vi "why_editsandweird.vi"() -> ()   [LabVIEW 2023]
uses:
  <vilib>/Analysis/NI_AALBase.lvlib
  <vilib>/DAQmx/read.llb/DAQmx Read (Analog 1D DBL NChan 1Samp).vi
  Supporting VIs/Logic states.ctl
  Supporting VIs/Motor states.ctl
  Supporting VIs/Axes indices.ctl
  <instrlib>/Arcus Driver 3.0.0/ArcusUsbComm/classes/Controller/_Controller.lvclass
  <instrlib>/Arcus Driver 3.0.0/ArcusUsbComm/common/controls/linear_direction.ctl
  Supporting VIs/Queue names.ctl
  <vilib>/addons/control/pid/NI_PID_pid.lvlib
  <vilib>/Utility/file.llb/Write Delimited Spreadsheet (string).vi
  <vilib>/Utility/file.llb/Write Delimited Spreadsheet (DBL).vi
  <vilib>/addons/control/pid/pid.llb/PID (DBL).vi
  <vilib>/DAQmx/configure/timing.llb/DAQmx Timing (Sample Clock).vi
  <vilib>/DAQmx/create/channels.llb/DAQmx Create Channel (AI-Voltage-Basic).vi
  <vilib>/Analysis/baseanly.llb/Vector x A.vi
  <vilib>/Analysis/baseanly.llb/A x Vector.vi
  Supporting VIs/Sampling frequency.ctl
panel:
  out "n":dbl format="%#_13g"
  in  "veloincrement":dbl format="%#_13g"
  in  "currentvelo":dbl format="%#_13g"
  in  "min velo":dbl
  in  "max velo":dbl
  in  "no of speedstops":dbl
  out "Steady State COFs":dbl[](array[numeric])
  out "Fixed amplitude Load":dbl(graph)=8.923720573303449
  in  "VISA resource name":refnum<visa-resource-name>
  out "Mean Estimated Friction Coefficient":dbl[](array[numeric])
  in  "Maximum COF Difference":i32=3000
  in  "Number of Previous Points":i32=3000
  out "Torque":dbl(graph)=-1.1532615270996815
  out "Sliding Distance (mm)":i32
  out "Angular Position":dbl
  in  "Initial Position":dbl
  in  "Track Radius (mm)":T1=100 items=["4 mm"=4, "6 mm"=6, "8 mm"=8, "10 mm"=10, "12 mm"=12, "14 mm"=14, "16 mm"=16, "18 mm"=18]
  out "Revolutions Completed":u8(slide) scale=0.0..10.0
  in  "STOP Rotating Motor":bool
  in  "Clockwise":bool
  in  "no of revs per velocity":i32
  out "Progress":dbl(slide) scale=0.0..100.0
  in  "Velocity":dbl
  in  "Units (0: microsteps)":u16(ring) items=["device speed units", "microns per second", "millimeters per second", "inches per second", "degrees per second"]
  in  "Microstep Size (0)":dbl
  in  "Wait [min]":dbl=30.0 format="%.2g"
  in  "Wait ?":bool=TRUE
  in  "Save file name":path=path "C:/Users/Egberts/Desktop/Tribometer/August 2020 Measurements/Tribometer/Late August 2020/test.txt"
  in  "PID gains":T2={"proportional gain (Kc)"=0.02, "integral time (Ti, min)"=0.1, "derivative time (Td, min)"=0.001} {"derivative time (Td, min)" format="%.3f"; "integral time (Ti, min)" format="%.3f"; "proportional gain (Kc)" format="%.3f"}
  in  "output range":cluster{"output high":dbl, "output low":dbl}={"output high"=2.0, "output low"=-2.0} {"output low" format="%.2f"; "output high" format="%.2f"}
  out "x-position":i32
  out "z-position":string
  in  "set zero":bool
  out "Correction loop":i32
  out "received P":i32
  out "Actual Load":dbl
  out "Correction [N]":dbl format="%.2f"
  out "correction [p]":dbl
  out "to PID":i32
  out "dt out (s)":dbl=0.25 format="%.3f"
  in  "Testing Load [N]":dbl=20.0
  in  "Wear cycles":i32=3000
  out "Manual control":bool
  in  "Approach":bool
  in  "DAQmx Device Name":tag="Dev1"
  in  "Out":bool
  in  "In":bool
  in  "Left":bool
  in  "Right":bool
  in  "Up":bool
  out "Estimated friction coefficient":dbl(graph)=-0.11599973982411911
  out "Smooth Force from Torque":dbl(graph)=-1.1532615270996815
  out "Smooth z":dbl(graph)=9.94193201509139
  out "Dequeued Data":dbl[](graph)=[9.378691263157721, 10.717600289594278, 8.438969804942502, 9.318124790458075, 8.681089909963866, 9.970529667476073, 10.834102440336615, 9.183821958337319, 9.334582664259113, 9.226213467034226, 10.238553338370796, 11.173780758664948, 8.690449558950064, 9.261606371512476, 8.790570665988898, 9.887706352746802, 11.038667014275244, 8.916330650848511, 9.104119720861869, 8.923720573303449]
  in  "ABORT":bool
  in  "Down":bool
  out "Aborted":bool
  out "Mean z":dbl[](array[numeric])
  out "Current reading":dbl[](array[numeric])
  in  "Averaging Level":i32=12
  out "Mean Force from Torque":dbl[](array[numeric])
  out "Completed":bool
  out "Testing":bool
  out "Approaching":bool
  in  "TARE":bool
  in  "Sampling frequency (rate)":T1=100 items=["1000 Hz"=1000, " 500 Hz"=500, " 250 Hz"=250, "100 Hz"=100, "50 Hz"=50, "10 Hz"=10, "1 Hz"=1]
  in  "Calibration file":path=path "C:/Users/Egberts/Desktop/ATI Industrial Automation/FT21774.cal"
  # "Counterclockwise"
  # "Originally used to measure \nthe amount of positions needed\nto perform fast approach"
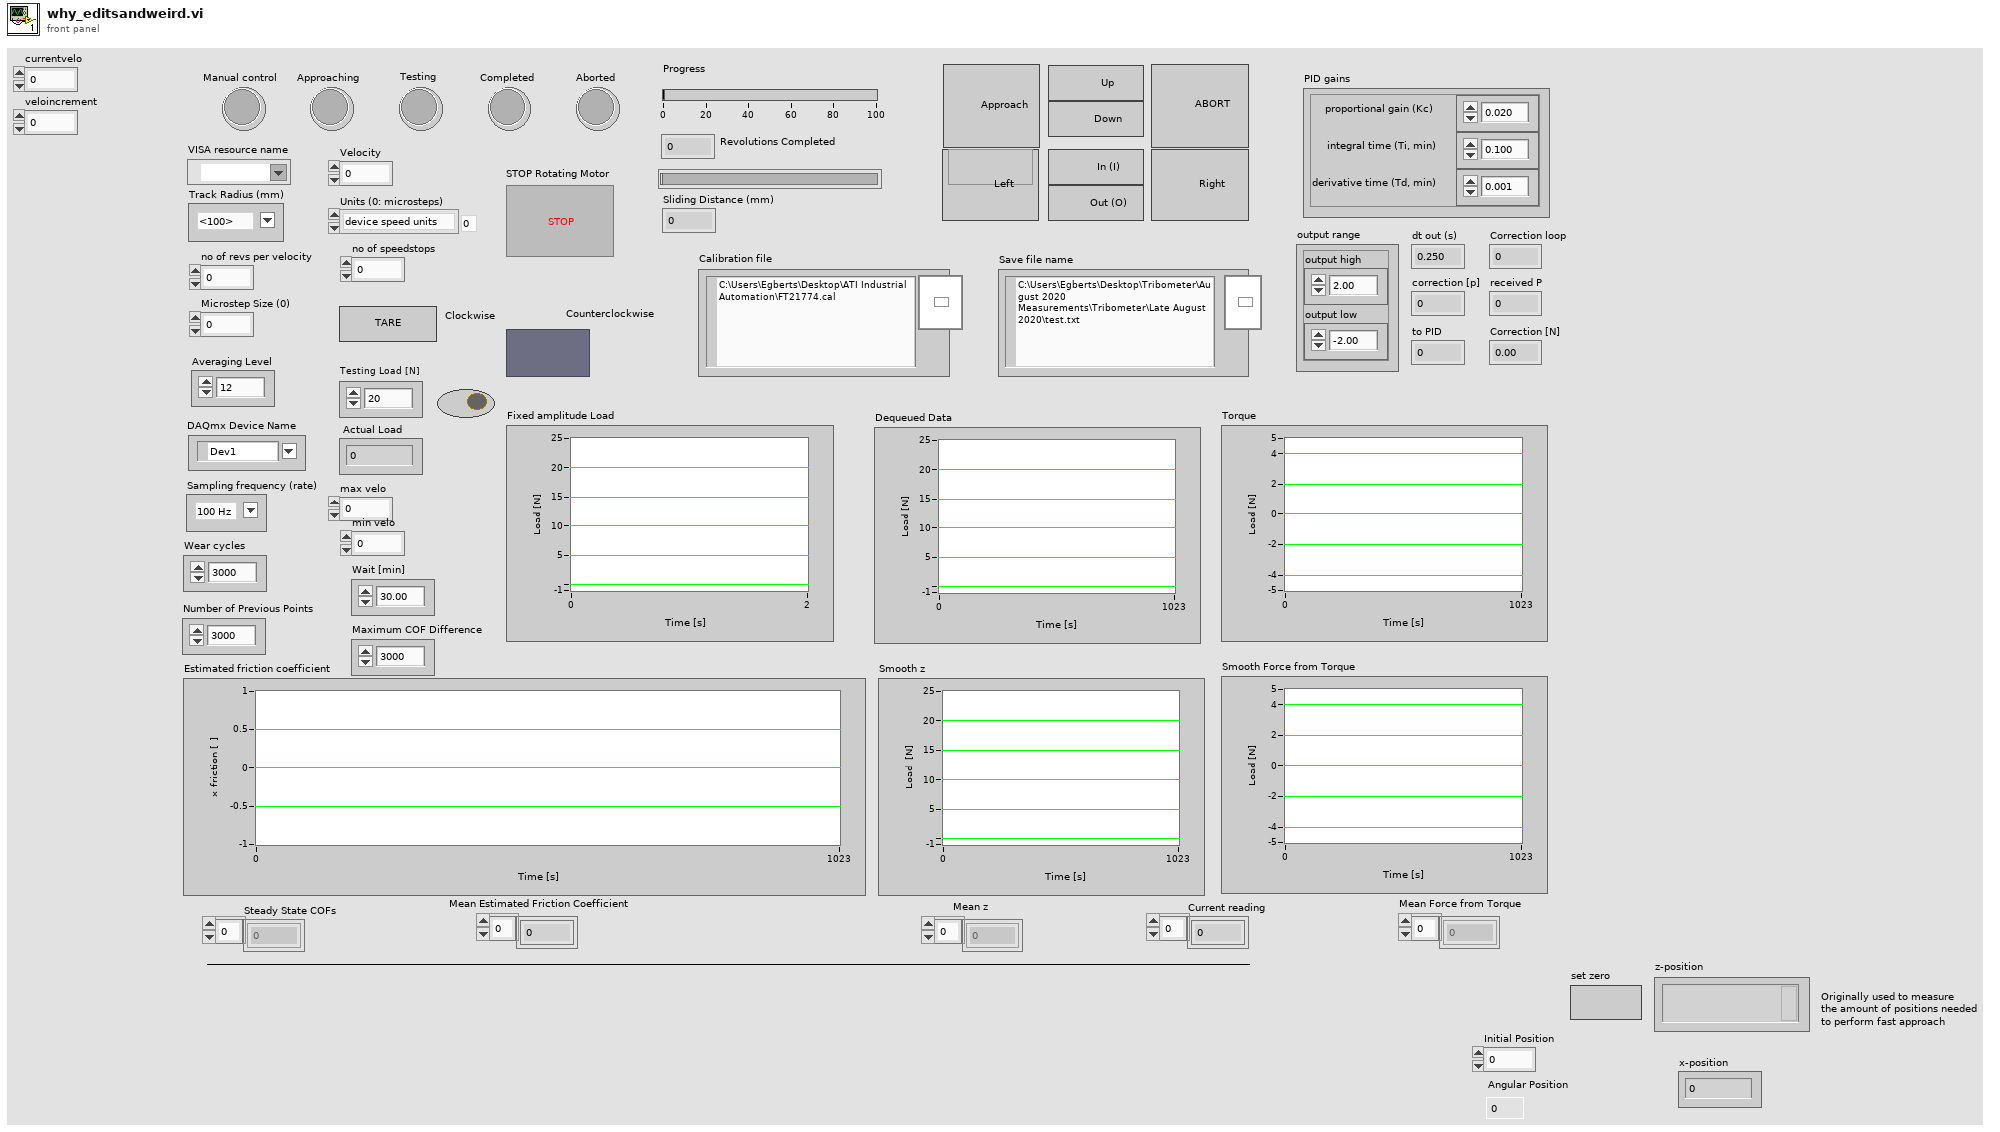
[diagram p1: front panel]
types:
  T1 = typedef "Sampling frequency.ctl" = u16
  T2 = cluster{"proportional gain (Kc)":dbl, "integral time (Ti, min)":dbl, "derivative time (Td, min)":dbl}
  T3 = typedef "Queue names.ctl" = enum16{"Cell queue name", "z-axis ref queue", "x-axis ref queue", "tangent-axis ref queue", "y-axis ref queue", "to PID", "Feedback"}
  T4 = typedef "Motor states.ctl" = enum16{"Initialize", "Manual control", "Approaching", "Testing", "Terminate"}
  T5 = typedef "Logic states.ctl" = enum16{"Initialize", "Process", "Terminate"}
  T6 = enum8{"Enabled", "Disabled", "Disabled and Grayed Out"}
  T7 = cluster{"queue out":refnum<queue>, "error out":errorcluster}
  T8 = cluster{"task out":refnum<k21>, "error out":errorcluster}
  T9 = cluster{"reference (out)":refnum<class "_Controller.lvclass">, "error out":errorcluster}
  T10 = typedef "Axes indices.ctl" = enum16{"y-axis", "x-axis", "z-axis"}
  T11 = cluster{"queue out":refnum<queue>, "queue out":refnum<queue>, "queue out":refnum<queue>}
  T12 = typedef "common.lvlib/linear_direction.ctl" = enum16{"POS (+)", "NEG (-)"}
  T13 = typedef "lveventtype.ctl" = enum32{"Null", "Timeout", "Annotation Menu Selection", "Annotation Menu Selection?", "App Instance Close", "App Instance Close?", "Autoscale Range Change", "Bookmark Info Change", "Cell Edit", "Cell Edit?", "Cursor Grab", "Cursor Grab?", "Cursor Menu Selection", "Cursor Menu Selection?", "Cursor Move", "Cursor Release", "Data Change", "Direction Change", "Display State Change", "Drag Ended", "Drag Enter", "Drag Leave", "Drag Over", "Drag Source Update", "Drag Starting", "Drag Starting?", "Drop", "Exec State Change", "Key Down", "Key Down?", "Key Repeat", "Key Repeat?", "Key Up", "Listbox Double Click", "Menu Activation?", "Menu Selection (App)", "Menu Selection? (App)", "Menu Selection (User)", "Mouse Down", "Mouse Down?", "Mouse Enter", "Mouse Leave", "Mouse Move", "Mouse Up", "Mouse Wheel", "NI Security User Change (App)", "Pane Size", "Panel Close", "Panel Close?", "Panel Resize", "Plot Attribute Change", "Scale Range Change", "Shortcut Menu Activation?", "Shortcut Menu Selection (App)", "Shortcut Menu Selection? (App)", "Shortcut Menu Selection (User)", "Tree Double Click", "Tree Drag", "Tree Drag?", "Tree Drop", "Tree Drop?", "Tree Item Close", "Tree Item Close?", "Tree Item Open", "Tree Item Open?", "User Event", "Value Change"}
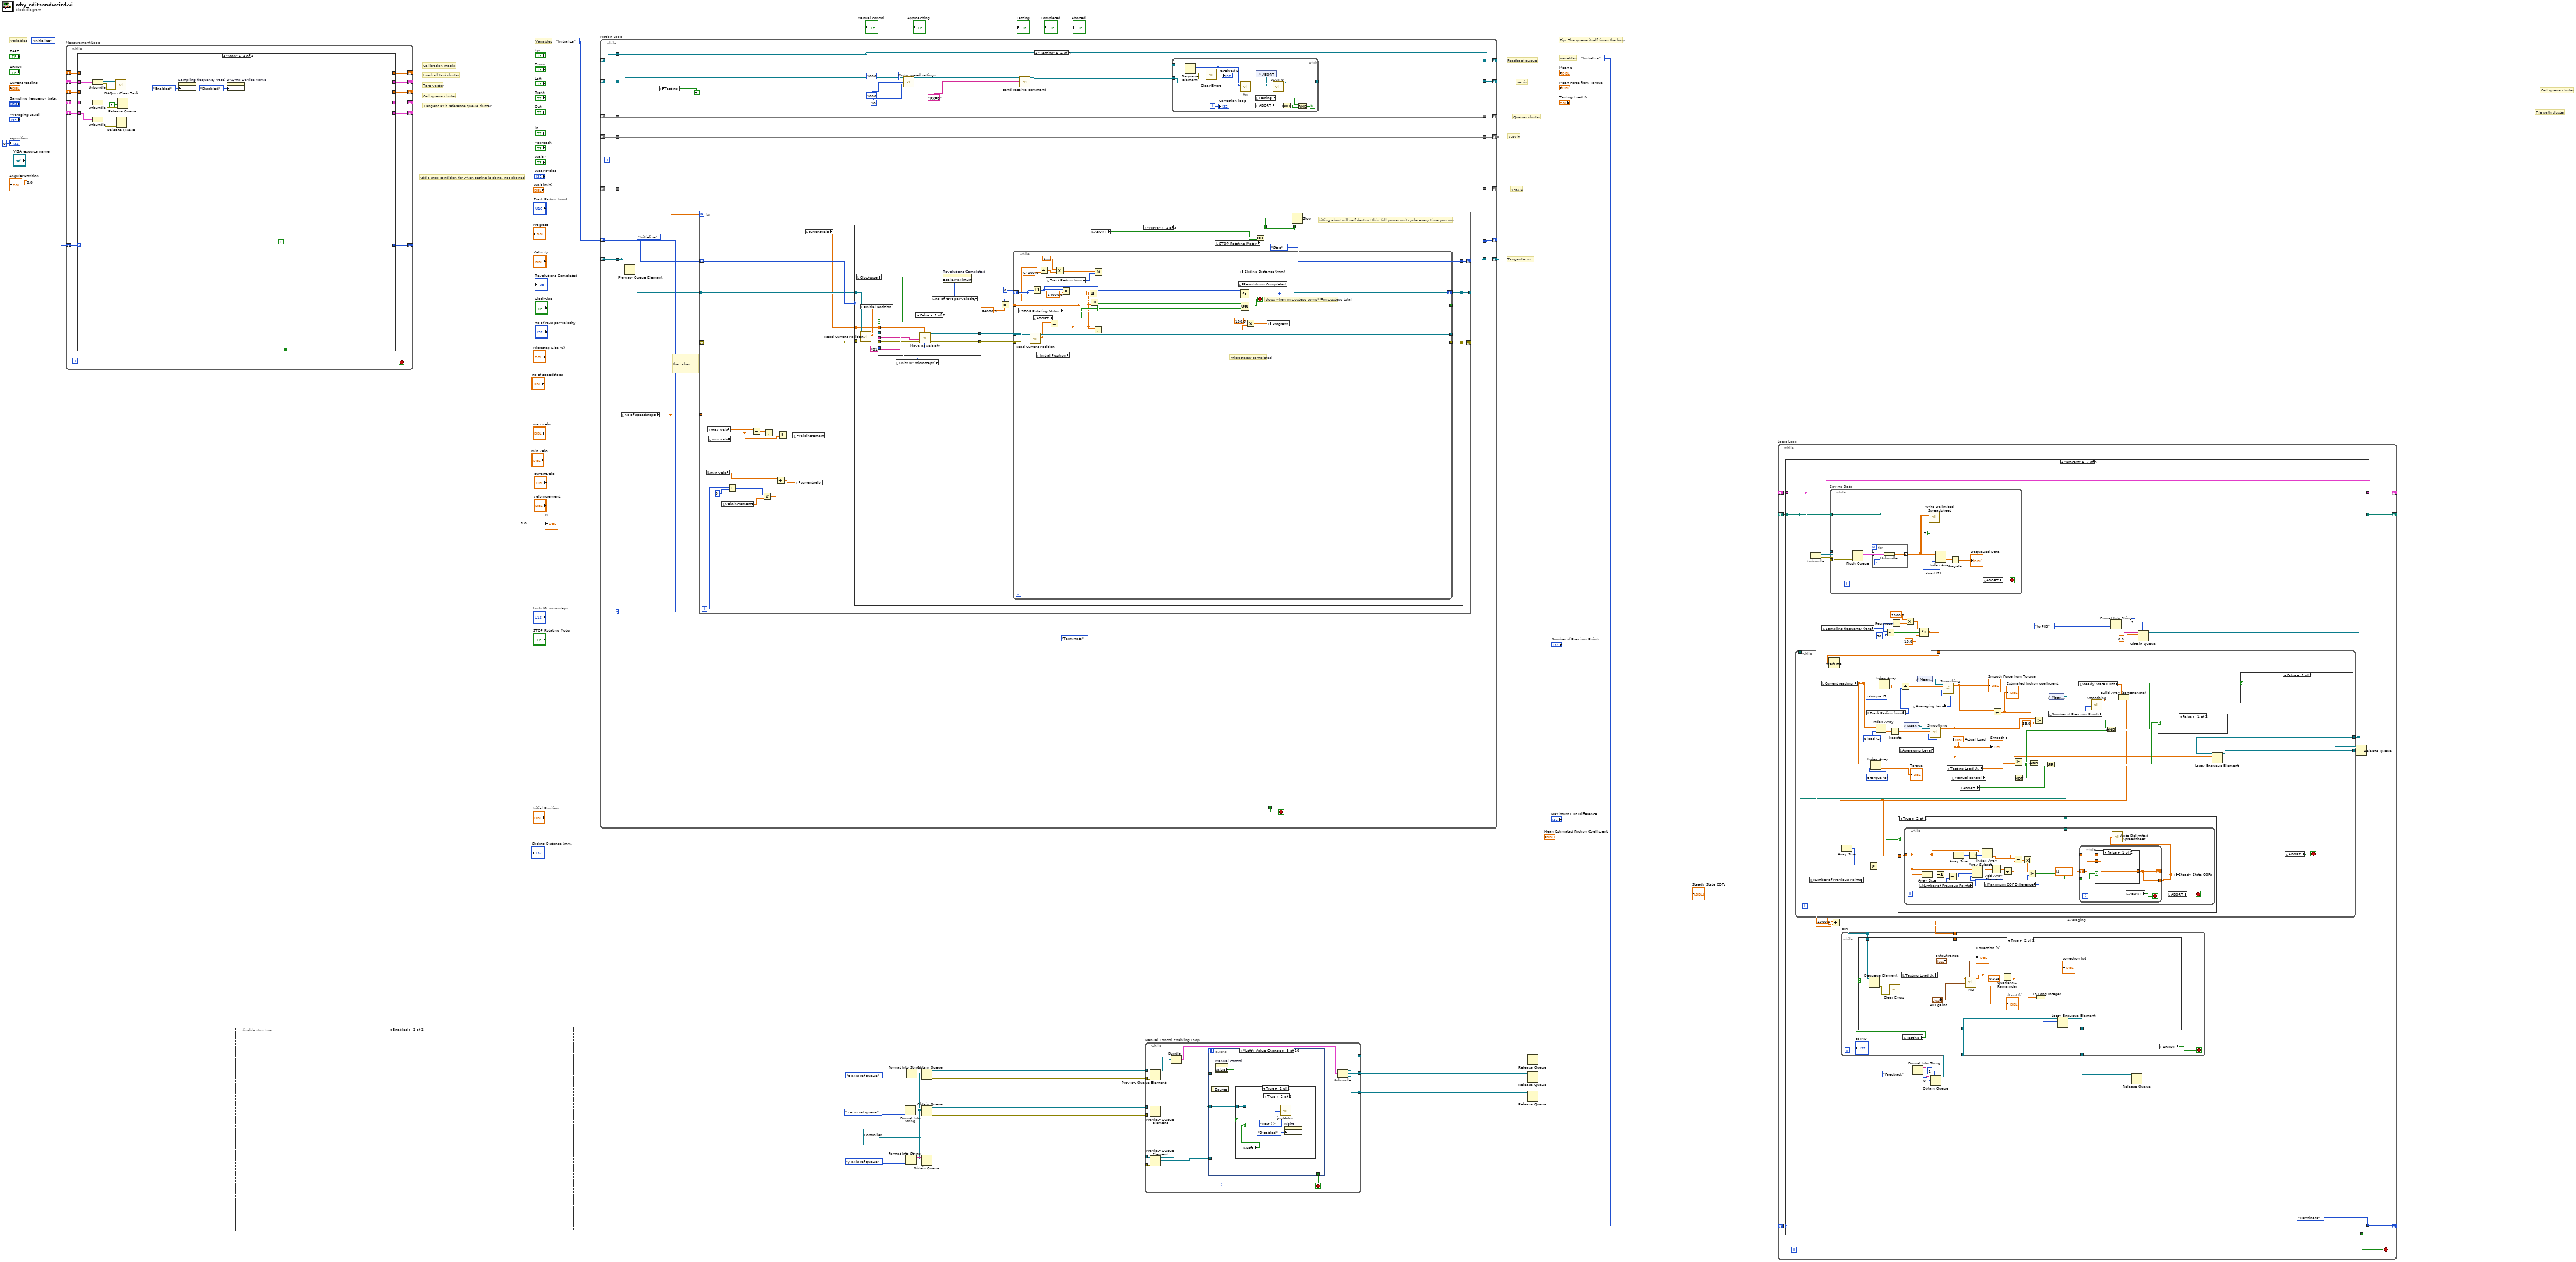
[diagram p0: block diagram]
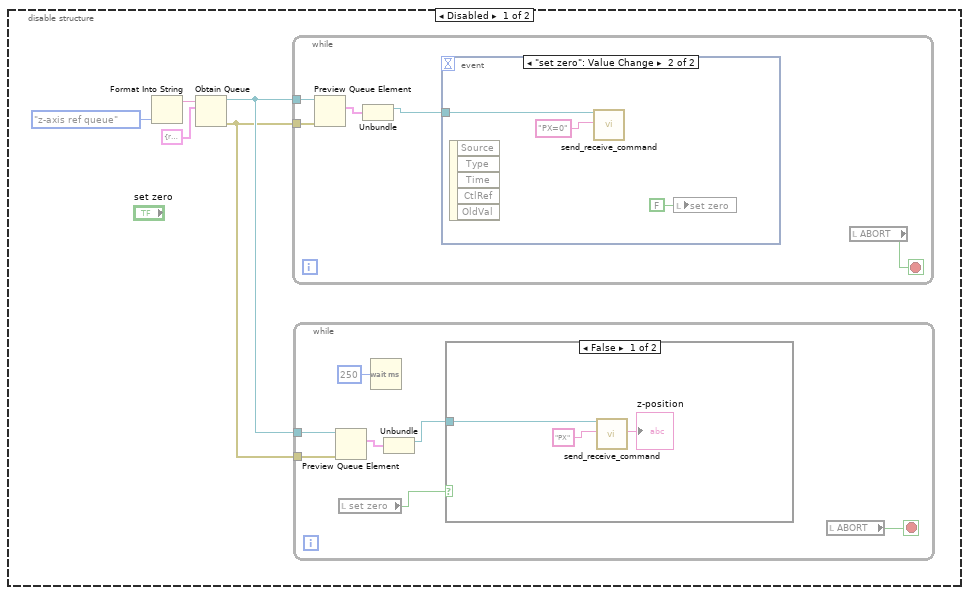
[diagram p2: hidden frame]
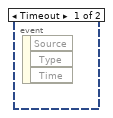
[diagram p4: hidden frame]
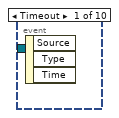
[diagram p5: hidden frame]
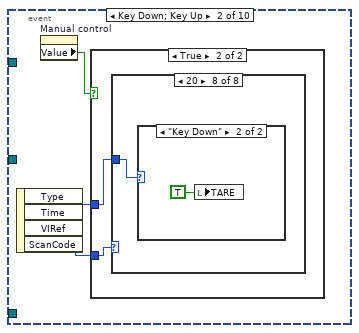
[diagram p6: hidden frame]
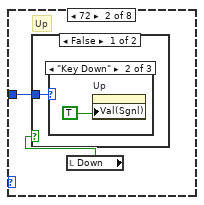
[diagram p9: hidden frame]
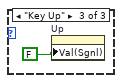
[diagram p11: hidden frame]
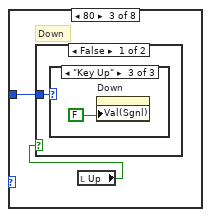
[diagram p13: hidden frame]
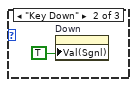
[diagram p15: hidden frame]
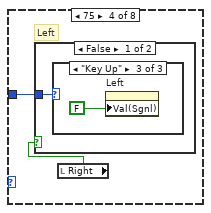
[diagram p17: hidden frame]
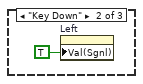
[diagram p19: hidden frame]
diagram:
  w3 = refnum<class "_Controller.lvclass"> refnum ("Controller in")
  # "Tangent-axis"
  # "Feedback queue"
  # "Queues cluster"
  # "Tangent axis reference queue cluster"
  # "Add a stop condition for when testing is done, not aborted"
  # "y-axis"
  # "x-axis"
  # "z-axis"
  # "Variables"
  # "Variables"
  # "File path cluster"
  # "Cell queue cluster"
  # "Tip: The queue itself times the loop"
  # "Variables"
  # "Cell queue cluster"
  # "Loadcell task cluster"
  # "Tare vector"
  # "Calibration matrix"
  n1 = while "Measurement Loop" {
    shift-right: [w34] -> _
    shift-left: enum16{"Initialize", "Tare", "Measure", "Stop"}."Initialize" ("Enum") -> [w35]
    shift-right: [w29] -> _
    shift-left: _ -> [w28]
    shift-right: [w33] -> _
    shift-left: _ -> [w31]
    shift-right: [w32] -> _
    shift-left: _ -> [w30]
    shift-right: [w25] -> _
    shift-left: _ -> [w26]
    shift-right: [w24] -> _
    shift-left: _ -> [w23]
    stop <- w27 stop-if-true
    n2 = case shown="\"Stop\"" w35 {
      tunnel: [w58 w83 w118 _] -> w34
      tunnel: [_ w90 _ _] -> w33
      tunnel: [w62 w82 w120 _] -> w32
      tunnel: w30 -> [_ w82 w120 w186]
      tunnel: w31 -> [_ _ w121 _]
      tunnel: [w61 w89 w119 _] -> w29
      tunnel: w28 -> [_ w89 w119 _]
      tunnel: [_ _ _ TRUE] -> w27
      tunnel: w26 -> [_ w77 w106 w183]
      tunnel: [w53 w77 w107 _] -> w25
      tunnel: [w42 w75 w114 _] -> w24
      tunnel: w23 -> [_ w75 w114 w177]
      frame "Initialize", Default {
        w66 = u16 10123 items=["Continous"=10123, "Finite"=10178, "Hardware Timed"=12522]  # Sample mode
        w73 = "N-M"  # Torque units
        w72 = "N"  # Force units
        n3 = local read "VISA resource name"() -> (w37:refnum<visa-resource-name>)
        n4 = property on="Sampling frequency (rate)" class="Ring (strict)"("DisabledEnum"=T6."Disabled" ("Disabled")) -> ()  [unwired: 2 in, 2 out]
        n5 = call "mxChannelList.vi"("First Channel"=0, "Number of Channels"=6, "DAQmx Device Name"="DAQmx Device Name") -> ("error out"=w68:errorcluster, "Channel List"=w69:string)  [unwired: 1 in]
        n6 = call <instrlib>:"Initialize.vi"("VISA resource name"=w37) -> ("VISA resource name out"=w36:refnum<visa-resource-name>)  [unwired: 9 in, 1 out]
        n7 = call "LoadCalibrationFromFile.vi"("User Torque Units"=w73, "User Force Units"=w72, "Cal File Path"="Calibration file") -> ("Calibration Matrix"=w61:dbl[][])  [unwired: 1 in, 3 out]
        n8 = property on="DAQmx Device Name" class="DAQmxName"("DisabledEnum"=T6."Disabled" ("Disabled")) -> ()  [unwired: 2 in, 2 out]
        n9 = Format Into String(Queue_names."Cell queue name" ("Enum")) -> (resulting string=w40:string)  [unwired: 3 in, 1 out]
        n10 = call-poly <vilib>:"DAQmx Create Virtual Channel.vi"("physical channels"=w69, "error in"=w68) -> ("task out"=w67:refnum<k21>, "error out"=w46:errorcluster)  [unwired: 12 in]
        n11 = local read "Sampling frequency (rate)"() -> (w52:T1)
        n12 = call-poly <vilib>:"DAQmx Timing.vi"("task/channels in"=w67, "sample mode"=w66, "rate"=w52) -> ("task out"=w65:refnum<k21>, "error out"=w64:errorcluster)  [unwired: 11 in]
        n13 = Format Into String(Queue_names."tangent-axis ref queue" ("Enum")) -> (resulting string=w38:string)  [unwired: 3 in, 1 out]
        n14 = call <vilib>:"DAQmx Start Task.vi"("task/channels in"=w65, "error in"=w64) -> ("task out"=w63:refnum<k21>, "error out"=w47:errorcluster)  [unwired: 12 in]
        n15 = Obtain Queue(name (unnamed)=w38, element data type=w36) -> (queue out=w44:refnum<queue>, error out=w43:errorcluster)  [unwired: 3 in, 1 out]
        n16 = Obtain Queue(name (unnamed)=w40, element data type=dbl[] []) -> (queue out=w54:refnum<queue>, error out=w48:errorcluster)  [unwired: 3 in, 1 out]
        n17 = local read "ABORT"() -> (w56:bool)
        n18 = Bundle("queue out"=w54, "error out"=w48) -> (w53:T7)  [unwired: 1 in]
        n19 = Bundle("queue out"=w44, "error out"=w43) -> (w42:T7)  [unwired: 1 in]
        n20 = Bundle("task out"=w63, "error out"=w47) -> (w62:T8)  [unwired: 1 in]
        n21 = Merge Errors(w43, w48, w47, w46) -> (w45:errorcluster)
        n22 = Compound Arithmetic op=OR(w45, w56) -> (w57:bool)
        n23 = Select(t=enum16{"Initialize", "Tare", "Measure", "Stop"}."Stop" ("Enum"), s=w57, f=enum16{"Initialize", "Tare", "Measure", "Stop"}."Tare" ("Enum")) -> (s? t:f=w58:enum16{"Initialize", "Tare", "Measure", "Stop"})
      }
      frame "Tare" {
        n24 = local read "Averaging Level"() -> (w76:i32)
        n25 = for {
          N: w76 -> [_]
          tunnel: w82 -> [w96]
          shift-right: [w98] -> w80
          shift-left: dbl[][] [] -> [w97]
          tunnel: [w95] -> w79
          tunnel: [FALSE] -> w78
          n26 = Unbundle(w96) -> ("task out"=w101:refnum<k21>, "error out"=w100:errorcluster)
          n27 = call-poly <vilib>:"DAQmx Read.vi"("task/channels in"=w101, "error in"=w100) -> ("data"=w99:dbl[], "error out"=w95:errorcluster)  [unwired: 11 in, 1 out]
          n28 = Build Array (concatenate)(w97, w99) -> (w98:dbl[][])
        }
        n29 = local write "TARE"(w78) -> ()
        n30 = Matrix Size(0:w80) -> (1:w91:i32)  [unwired: 1 out]
        n31 = Reciprocal(x=w91) -> (1/x=w92:dbl)
        n32 = Unbundle By Name(w79) -> ("status"=w84:bool)
        n33 = local read "ABORT"() -> (w85:bool)
        n34 = Initialize Array(w92, w91) -> (w93:dbl[])
        n35 = Or(x=w84, y=w85) -> (x .or. y?=w88:bool)
        n36 = call-poly <vilib>:"A x B.vi"("Matrix A"=w80, "Vector V'"=w93) -> ("V' x A"=w90:dbl[])  [unwired: 1 out]
        n37 = Select(t=enum16{"Initialize", "Tare", "Measure", "Stop"}."Stop" ("Enum"), s=w88, f=enum16{"Initialize", "Tare", "Measure", "Stop"}."Measure" ("Enum")) -> (s? t:f=w83:enum16{"Initialize", "Tare", "Measure", "Stop"})
      }
      frame "Measure" {
        n38 = Unbundle(w114) -> ("queue out"=w103:refnum<queue>, "error out"=w102:errorcluster)
        n39 = Unbundle(w106) -> ("queue out"=w105:refnum<queue>, "error out"=w104:errorcluster)
        n40 = Unbundle(w114) -> ("queue out"=w113:refnum<queue>, "error out"=w112:errorcluster)
        n41 = Unbundle(w120) -> ("task out"=w111:refnum<k21>, "error out"=w110:errorcluster)
        n42 = while {
          tunnel: w121 -> [w162]
          tunnel: w119 -> [w154]
          tunnel: [w152] -> w115
          tunnel: w113 -> [w145]
          tunnel: w112 -> [w144]
          tunnel: w111 -> [w143]
          tunnel: w110 -> [w142]
          tunnel: [w141] -> w109
          tunnel: [w140] -> w108
          tunnel: w105 -> [w139]
          tunnel: w104 -> [w138]
          stop <- w157 stop-if-true
          w159 = u16 2 items=["x-load", "y-load", "z-load", "x-torque", "y-torque", "z-torque"]
          n43 = Get Queue Status(queue=w145, error in (no error)=w144) -> (# elements in queue=w149:i32)  [unwired: 1 in, 7 out]
          n44 = local read "Testing"() -> (w148:bool)
          n45 = call-poly <vilib>:"DAQmx Read.vi"("task/channels in"=w143, "error in"=w142) -> ("data"=w155:dbl[], "error out"=w153:errorcluster)  [unwired: 11 in, 1 out]
          n46 = Not Equal To 0?(x=w149) -> (x != 0?=w147:bool)
          n47 = And(x=w147, y=w148) -> (x .and. y?=w146:bool)
          n48 = Subtract(x=w155, y=w162) -> (x-y=w161:dbl[])
          n49 = call-poly <vilib>:"A x B.vi"("Vector"=w161, "A"=w154) -> ("A x Vector"=w150:dbl[])  [unwired: 1 out]
          n50 = case shown="True" w146 {
            tunnel: [FALSE ("status") w174] -> w151
            tunnel: w150 -> [_ w173]
            tunnel: w139 -> [w164 w171]
            tunnel: w138 -> [w163 w170]
            tunnel: [w164 w169] -> w141
            tunnel: [w163 w168] -> w140
            frame False {
            }
            frame True {
              n51 = local read "Angular Position"() -> (w166:dbl)
              n52 = To Long Integer(number=w166) -> (32bit integer=w167:i32)
              n53 = Build Array (concatenate)(w173, w167) -> (w172:dbl[])
              n54 = Enqueue Element(queue=w171, element=w172, error in (no error)=w170) -> (queue out=w169:refnum<queue>, error out=w168:errorcluster)  [unwired: 1 in, 1 out]
              n55 = Unbundle By Name(w168) -> ("status"=w174:bool)
            }
          }
          n56 = local write "Current reading"(w150) -> ()
          n57 = Index Array(array=w150, index=w159) -> (element=w160:dbl)
          n58 = Negate(x=w160) -> (-x=→"Fixed amplitude Load":dbl)
          n59 = local read "TARE"() -> (w152:bool)
          n60 = Unbundle By Name(w153) -> ("status"=w156:bool)
          n61 = local read "ABORT"() -> (w158:bool)
          n62 = Compound Arithmetic op=OR(w151, w152, w158, w156) -> (w157:bool)
        }
        n63 = while {
          tunnel: w103 -> [w123]
          tunnel: w102 -> [w122]
          stop <- w125 stop-if-true
          n64 = local read "Testing"() -> (w129:bool)
          n65 = Get Queue Status(queue=w123, error in (no error)=w122) -> (queue out=w127:refnum<queue>, # elements in queue=w131:i32)  [unwired: 1 in, 6 out]
          n66 = Not Equal To 0?(x=w131) -> (x != 0?=w130:bool)
          n67 = And(x=w130, y=w129) -> (x .and. y?=w128:bool)
          n68 = case shown="True" w128 {
            tunnel: w127 -> [_ w135]
            frame False {
            }
            frame True {
              n69 = Preview Queue Element(queue=w135) -> (element=w134:refnum<visa-resource-name>)  [unwired: 2 in, 3 out]
              n70 = call <instrlib>:"Read Current Position.vi"("Device and Axis"="PX", "VISA resource name"=w134) -> ("VISA resource name out"=w132:refnum<visa-resource-name>)  [unwired: 7 in, 2 out]
              n71 = Decimal String To Number(string=w132) -> (number=w136:i32)  [unwired: 2 in, 1 out]
              n72 = local write "Angular Position"(w136) -> ()
            }
          }
          n73 = local read "ABORT"() -> (w126:bool)
          n74 = local read "TARE"() -> (w124:bool)
          n75 = Or(x=w126, y=w124) -> (x .or. y?=w125:bool)
        }
        n76 = Select(t=enum16{"Initialize", "Tare", "Measure", "Stop"}."Tare" ("Enum"), s=w115, f=enum16{"Initialize", "Tare", "Measure", "Stop"}."Stop" ("Enum")) -> (s? t:f=w118:enum16{"Initialize", "Tare", "Measure", "Stop"})
        n77 = Bundle("queue out"=w109, "error out"=w108) -> (w107:T7)  [unwired: 1 in]
      }
      frame "Stop" {
        n78 = Unbundle(w186) -> ("task out"=w185:refnum<k21>, "error out"=w184:errorcluster)
        n79 = Unbundle(w183) -> ("queue out"=w182:refnum<queue>, "error out"=w181:errorcluster)
        n80 = Unbundle(w177) -> ("queue out"=w176:refnum<queue>, "error out"=w175:errorcluster)
        n81 = call <vilib>:"DAQmx Clear Task.vi"("task in"=w185, "error in"=w184) -> ()  [unwired: 13 in, 1 out]
        n82 = Release Queue(queue=w176, error in (no error)=w175) -> ()  [unwired: 1 in, 3 out]
        n83 = Release Queue(queue=w182, force destroy? (F)=FALSE, error in (no error)=w181) -> ()  [unwired: 3 out]
        n84 = property on="Sampling frequency (rate)" class="Ring (strict)"("DisabledEnum"=T6."Enabled" ("Disabled")) -> ()  [unwired: 2 in, 2 out]
        n85 = property on="DAQmx Device Name" class="DAQmxName"("DisabledEnum"=T6."Disabled" ("Disabled")) -> ()  [unwired: 2 in, 2 out]
      }
    }
  }
  n86 = disable-structure shown="Enabled" {
    frame Disabled {
      n87 = Format Into String(Queue_names."z-axis ref queue" ("Enum")) -> (resulting string=w191:string)  [unwired: 3 in, 1 out]
      n88 = Obtain Queue(name (unnamed)=w191, element data type=T9 {"reference (out)"=refnum, "error out"={"status"=FALSE, "code"=0, "source"=""}} ("output cluster")) -> (queue out=w189:refnum<queue>, error out=w188:errorcluster)  [unwired: 3 in, 1 out]
      n89 = while {
        tunnel: w189 -> [w207]
        tunnel: w188 -> [w206]
        stop <- w203 stop-if-true
        n90 = Preview Queue Element(queue=w207, error in (no error)=w206) -> (element=w205:T9)  [unwired: 1 in, 3 out]
        n91 = Unbundle(w205) -> ("reference (out)"=w204:refnum<class "_Controller.lvclass">)  [unwired: 1 out]
        n92 = event shown="[1] \"set zero\": Value Change" {
          selector: _ -> [_ _]
          dyn-events: _ -> [_ _]
          timeout: _ -> [_ _]
          tunnel: w204 -> [_ w210]
          event Timeout {
            n93 = event-data() -> ()  [unwired: 1 in, 3 out]
          }
          event "set zero": Value Change {
            n94 = event-data() -> ()  [unwired: 1 in, 5 out]
            n95 = call <instrlib>:"send_receive_command.vi"("reference (in)"=w210, "ASCII Command (in)"="PX=0") -> ()  [unwired: 13 in, 5 out]
            n96 = local write "set zero"(FALSE ("set zero")) -> ()
          }
        }
        n97 = local read "ABORT"() -> (w203:bool)
      }
      n98 = while {
        tunnel: w189 -> [w196]
        tunnel: w188 -> [w195]
        stop <- w198 stop-if-true
        n99 = Preview Queue Element(queue=w196, error in (no error)=w195) -> (element=w197:T9)  [unwired: 1 in, 3 out]
        n100 = local read "set zero"() -> (w193:bool)
        n101 = Wait (ms)(milliseconds to wait=u32 250) -> ()  [unwired: 1 out]
        n102 = Unbundle(w197) -> ("reference (out)"=w194:refnum<class "_Controller.lvclass">)  [unwired: 1 out]
        n103 = case shown="False" w193 {
          tunnel: w194 -> [w201 _]
          frame False {
            n104 = call <instrlib>:"send_receive_command.vi"("reference (in)"=w201, "ASCII Command (in)"="PX") -> ("response (out)"=→"z-position":string)  [unwired: 13 in, 4 out]
          }
          frame True {
          }
        }
        n105 = local read "ABORT"() -> (w198:bool)
      }
    }
    frame Enabled {
    }
  }
  n106 = while "Motion Loop" {
    shift-right: [w224] -> _
    shift-left: Motor_states."Initialize" -> [w225]
    shift-right: [w216] -> _
    shift-left: _ -> [w223]
    shift-right: [w215] -> _
    shift-left: _ -> [w213]
    shift-right: [w214] -> _
    shift-left: _ -> [w222]
    shift-right: [w220] -> _
    shift-left: _ -> [w219]
    shift-right: [w218] -> _
    shift-left: _ -> [w217]
    shift-right: [w212] -> _
    shift-left: _ -> [w211]
    stop <- w221 stop-if-true
    n107 = case shown="\"Testing\"" w225 {
      tunnel: [Motor_states."Manual control" w295 w317 Motor_states."Terminate" _] -> w224
      tunnel: w223 -> [_ w280 w308 w367 w494]
      tunnel: w222 -> [_ w276 w310 w365 w492]
      tunnel: [_ _ _ _ w500] -> w221
      tunnel: [w244 w282 w313 w372 _] -> w220
      tunnel: w219 -> [_ w282 w313 w372 w499]
      tunnel: [w239 w281 w312 w371 _] -> w218
      tunnel: w217 -> [_ w281 w312 w371 w495]
      tunnel: [w238 w279 w311 w366 _] -> w216
      tunnel: [w237 w277 w305 w364 _] -> w215
      tunnel: [w236 w275 w310 w365 _] -> w214
      tunnel: w213 -> [_ w278 w306 w364 w493]
      tunnel: [w229 w274 w304 w361 _] -> w212
      tunnel: w211 -> [_ w274 w304 w361 _]
      frame "Initialize" {
        w226 = TRUE
        w235 = FALSE ("Approach")
        n108 = local write "Testing"(w235) -> ()
        n109 = local write "Aborted"(w235) -> ()
        n110 = local write "Approach"(w235) -> ()
        n111 = local write "Approaching"(w235) -> ()
        n112 = local write "Completed"(w235) -> ()
        n113 = local write "Progress"(0 ("Test Progress")) -> ()
        n114 = local read "VISA resource name"() -> (w231:refnum<visa-resource-name>)
        n115 = call <instrlib>:"initialize.vi"("device_index (in) [0=def]"=Axes_indices."x-axis", "clear_buffer? (T)"=w226) -> ("reference (out)"=w268:refnum<class "_Controller.lvclass">)  [unwired: 16 in, 1 out]
        n116 = call <instrlib>:"initialize.vi"("device_index (in) [0=def]"=Axes_indices."y-axis", "clear_buffer? (T)"=w226) -> ("reference (out)"=w267:refnum<class "_Controller.lvclass">)  [unwired: 16 in, 1 out]
        n117 = call <instrlib>:"initialize.vi"("device_index (in) [0=def]"=Axes_indices."z-axis", "clear_buffer? (T)"=w226) -> ("reference (out)"=w269:refnum<class "_Controller.lvclass">)  [unwired: 16 in, 1 out]
        n118 = call <instrlib>:"send_receive_command.vi"("reference (in)"=w268, "ASCII Command (in)"="SR0=0") -> ("reference (out)"=w262:refnum<class "_Controller.lvclass">)  [unwired: 13 in, 4 out]
        n119 = call <instrlib>:"send_receive_command.vi"("reference (in)"=w267, "ASCII Command (in)"="SR0=0") -> ("reference (out)"=w263:refnum<class "_Controller.lvclass">)  [unwired: 13 in, 4 out]
        n120 = call <instrlib>:"send_receive_command.vi"("reference (in)"=w269, "ASCII Command (in)"="SR0=0") -> ("reference (out)"=w261:refnum<class "_Controller.lvclass">)  [unwired: 13 in, 4 out]
        n121 = call <instrlib>:"Initialize.vi"("VISA resource name"=w231) -> ("VISA resource name out"=w227:refnum<visa-resource-name>)  [unwired: 9 in, 1 out]
        n122 = call <instrlib>:"send_receive_command.vi"("reference (in)"=w262, "ASCII Command (in)"="INC") -> ("reference (out)"=w237:refnum<class "_Controller.lvclass">)  [unwired: 13 in, 4 out]
        n123 = call <instrlib>:"send_receive_command.vi"("reference (in)"=w263, "ASCII Command (in)"="INC") -> ("reference (out)"=w236:refnum<class "_Controller.lvclass">)  [unwired: 13 in, 4 out]
        n124 = call <instrlib>:"send_receive_command.vi"("reference (in)"=w261, "ASCII Command (in)"="INC") -> ("reference (out)"=w238:refnum<class "_Controller.lvclass">)  [unwired: 13 in, 4 out]
        n125 = Format Into String(Queue_names."tangent-axis ref queue" ("Enum")) -> (resulting string=w232:string)  [unwired: 3 in, 1 out]
        n126 = Obtain Queue(name (unnamed)=w232, element data type=w227) -> (queue out=w230:refnum<queue>, error out=w228:errorcluster)  [unwired: 3 in, 1 out]
        n127 = Enqueue Element(queue=w230, element=w227, error in (no error)=w228) -> (queue out=w229:refnum<queue>)  [unwired: 1 in, 2 out]
        n128 = Format Into String(Queue_names."Feedback" ("Enum")) -> (resulting string=w243:string)  [unwired: 3 in, 1 out]
        n129 = Format Into String(Queue_names."y-axis ref queue" ("Enum")) -> (resulting string=w251:string)  [unwired: 3 in, 1 out]
        n130 = Format Into String(Queue_names."x-axis ref queue" ("Enum")) -> (resulting string=w252:string)  [unwired: 3 in, 1 out]
        n131 = Format Into String(Queue_names."z-axis ref queue" ("Enum")) -> (resulting string=w253:string)  [unwired: 3 in, 1 out]
        n132 = Obtain Queue(max queue size (-1, unlimited)=1, name (unnamed)=w243, element data type=0) -> (queue out=w239:refnum<queue>)  [unwired: 2 in, 2 out]
        n133 = Obtain Queue(name (unnamed)=w251, element data type=w236) -> (queue out=w258:refnum<queue>, error out=w257:errorcluster)  [unwired: 3 in, 1 out]
        n134 = Obtain Queue(name (unnamed)=w252, element data type=w237) -> (queue out=w259:refnum<queue>)  [unwired: 3 in, 2 out]
        n135 = Obtain Queue(name (unnamed)=w253, element data type=w238) -> (queue out=w260:refnum<queue>)  [unwired: 3 in, 2 out]
        n136 = Enqueue Element(queue=w259, element=w237) -> (queue out=w246:refnum<queue>)  [unwired: 2 in, 2 out]
        n137 = Enqueue Element(queue=w258, element=w236, error in (no error)=w257) -> (queue out=w245:refnum<queue>)  [unwired: 1 in, 2 out]
        n138 = Enqueue Element(queue=w260, element=w238) -> (queue out=w247:refnum<queue>)  [unwired: 2 in, 2 out]
        n139 = Bundle("queue out"=w247, "queue out"=w246, "queue out"=w245) -> (w244:T11)  [unwired: 1 in]
      }
      frame "Manual control" {
        n140 = while {
          tunnel: [w301] -> w284
          stop <- w300 stop-if-true
          n141 = Wait Until Next ms Multiple(millisecond multiple=u32 150) -> ()  [unwired: 1 out]
          n142 = local read "Approach"() -> (w302:bool)
          n143 = local read "ABORT"() -> (w301:bool)
          n144 = Or(x=w302, y=w301) -> (x .or. y?=w300:bool)
        }
        n145 = local write "Manual control"(TRUE ("Manual control")) -> ()
        n146 = call "Motor speed settings.vi"("reference (in)"=w276, "HSPD"=13000 ("High Speed"), "LSPD"=100 ("Low Speed"), "ACC"=250 ("Acceleration Time")) -> ("reference (out)"=w275:refnum<class "_Controller.lvclass">)  [unwired: 10 in, 1 out]
        n147 = call "Motor speed settings.vi"("reference (in)"=w280, "HSPD"=13000 ("High Speed"), "LSPD"=100 ("Low Speed"), "ACC"=250 ("Acceleration Time")) -> ("reference (out)"=w279:refnum<class "_Controller.lvclass">)  [unwired: 10 in, 1 out]
        n148 = call "Motor speed settings.vi"("reference (in)"=w278, "HSPD"=13000 ("High Speed"), "LSPD"=100 ("Low Speed"), "ACC"=250 ("Acceleration Time")) -> ("reference (out)"=w277:refnum<class "_Controller.lvclass">)  [unwired: 10 in, 1 out]
        n149 = case shown="False" w284 {
          tunnel: [FALSE TRUE] -> w283
          frame False {
          }
          frame True {
          }
        }
        n150 = local write "Manual control"(w283) -> ()
        n151 = Select(t=Motor_states."Terminate", s=w284, f=Motor_states."Approaching") -> (s? t:f=w295:T4)
      }
      frame "Approaching" {
        n152 = flat-sequence {
          tunnel: w308 -> [w321]
          tunnel: [w320] -> w307
          tunnel: [w330] -> w309
          tunnel: w307 -> [w329]
          tunnel: w306 -> [w328]
          tunnel: [w327] -> w305
          frame #0 {
            n153 = local read "Wait ?"() -> (w322:bool)
            n154 = case shown="True" w322 {
              tunnel: w321 -> [w323 w324]
              tunnel: [w323 w324] -> w320
              frame False {
              }
              frame True {
                n155 = control-ref of="ABORT"() -> (w326:refnum<vi>)
                n156 = control-ref of="Wait [min]"() -> (w325:refnum<vi>)
                n157 = call "PASSIVATE.vi"("reference"=w325, "Boolean in"=w326) -> ()  [unwired: 1 in]
              }
            }
          }
          frame #1 {
            n158 = call "Motor speed settings.vi"("reference (in)"=w329, "HSPD"=22000 ("High Speed"), "LSPD"=1000 ("Low Speed"), "ACC"=500 ("Acceleration Time")) -> ("reference (out)"=w339:refnum<class "_Controller.lvclass">)  [unwired: 10 in, 1 out]
            n159 = call "Motor speed settings.vi"("reference (in)"=w328, "HSPD"=1000, "LSPD"=1000, "ACC"=10) -> ("reference (out)"=w346:refnum<class "_Controller.lvclass">)  [unwired: 10 in, 1 out]
            n160 = local read "Track Radius (mm)"() -> (w348:T1)
            n161 = control-ref of="ABORT"() -> (w340:refnum<vi>)
            n162 = call "Xn.vi"("Position"=55000, "_Controller in"=w339) -> ("_Controller out"=w341:refnum<class "_Controller.lvclass">)  [unwired: 8 in, 1 out]
            n163 = call "WAIT 0.vi"("reference"=w340, "_Controller in"=w341) -> ("_Controller out"=w338:refnum<class "_Controller.lvclass">)  [unwired: 7 in, 2 out]
            n164 = control-ref of="ABORT"() -> (w350:refnum<vi>)
            n165 = Multiply(x=w348, y=800) -> (x*y=w349:i32)
            n166 = call "Xn.vi"("Position"=w349, "_Controller in"=w346) -> ("_Controller out"=w347:refnum<class "_Controller.lvclass">)  [unwired: 8 in, 1 out]
            n167 = call "Motor speed settings.vi"("reference (in)"=w338, "HSPD"=100 ("High Speed"), "LSPD"=100 ("Low Speed"), "ACC"=10 ("Acceleration Time")) -> ("reference (out)"=w330:refnum<class "_Controller.lvclass">)  [unwired: 10 in, 1 out]
            n168 = call "WAIT 0.vi"("reference"=w350, "_Controller in"=w347) -> ("_Controller out"=w327:refnum<class "_Controller.lvclass">)  [unwired: 7 in, 2 out]
          }
        }
        n169 = local write "Approaching"(TRUE ("Approaching")) -> ()
        n170 = while {
          tunnel: [w353] -> w311
          tunnel: [w356] -> w316
          tunnel: [w355] -> w314
          tunnel: w309 -> [w351]
          stop <- w355 continue-if-true
          n171 = local read "Approaching"() -> (w359:bool)
          n172 = local read "ABORT"() -> (w356:bool)
          n173 = control-ref of="ABORT"() -> (w352:refnum<vi>)
          n174 = call "Xn.vi"("Position"=15, "_Controller in"=w351) -> ("_Controller out"=w354:refnum<class "_Controller.lvclass">)  [unwired: 8 in, 1 out]
          n175 = Not(x=w356) -> (.not. x?=w357:bool)
          n176 = And(x=w359, y=w357) -> (x .and. y?=w355:bool)
          n177 = call "WAIT 0.vi"("reference"=w352, "_Controller in"=w354) -> ("_Controller out"=w353:refnum<class "_Controller.lvclass">)  [unwired: 7 in, 2 out]
        }
        n178 = Select(t=Motor_states."Terminate", s=w316, f=Motor_states."Testing") -> (s? t:f=w317:T4)
        n179 = local write "Approaching"(w314) -> ()
      }
      frame "Testing" {
        # "the zaber"
        n180 = local read "no of speedstops"() -> (w360:dbl)
        n181 = Preview Queue Element(queue=w361) -> (element=w362:refnum<visa-resource-name>)  [unwired: 2 in, 3 out]
        n182 = local write "Testing"(TRUE ("Testing")) -> ()
        n183 = for {
          N: w360 -> [_]
          shift-right: [w397] -> _
          shift-left: enum16{"Initialize", "Move", "Stop"}."Initialize" -> [w398]
          shift-right: [w396] -> _
          shift-left: _ -> [w395]
          tunnel: w362 -> [w394]
          tunnel: [w393] -> _
          tunnel: w360 -> [w385]
          i -> [w382]
          # "hitting abort will self destruct this. full power unit cycle every time you run."
          n184 = local read "min velo"() -> (w384:dbl)
          n185 = local read "max velo"() -> (w391:dbl)
          n186 = local read "min velo"() -> (w388:dbl)
          n187 = local read "veloincrement"() -> (w380:dbl)
          n188 = Add(x=w382, y=0) -> (x+y=w381:i32)
          n189 = Subtract(x=w391, y=w388) -> (x-y=w390:dbl)
          n190 = Multiply(x=w381, y=w380) -> (x*y=w379:dbl)
          n191 = Divide(x=w390, y=w385) -> (x/y=w389:dbl)
          n192 = Add(x=w384, y=w379) -> (x+y=w378:dbl)
          n193 = Add(x=w389, y=w388) -> (x+y=w387:dbl)
          n194 = local write "veloincrement"(w387) -> ()
          n195 = local write "currentvelo"(w378) -> ()
          n196 = local read "currentvelo"() -> (w392:dbl)
          n197 = case shown="\"Move\"" w398 {
            tunnel: [enum16{"Initialize", "Move", "Stop"}."Move" enum16{"Initialize", "Move", "Stop"}."Stop" _] -> w397
            tunnel: [w404 w415 _] -> w396
            tunnel: w395 -> [_ w416 w472]
            tunnel: [w401 w406 TRUE] -> _
            tunnel: w394 -> [w399 w411 w470]
            tunnel: [w400 w410 _] -> w393
            tunnel: w392 -> [_ w407 _]
            tunnel: [_ w406 _] -> w386
            frame "Initialize", Default {
              n198 = call <instrlib>:"Initialize.vi"("VISA resource name"=w399) -> ("error out"=w404:errorcluster, "VISA resource name out"=w400:refnum<visa-resource-name>)  [unwired: 9 in]
              n199 = local read "STOP Rotating Motor"() -> (w402:bool)
              n200 = local read "ABORT"() -> (w403:bool)
              n201 = Or(x=w403, y=w402) -> (x .or. y?=w401:bool)
            }
            frame "Move" {
              n202 = local read "Clockwise"() -> (w426:bool)
              n203 = call <instrlib>:"Read Current Position.vi"("error in (no error)"=w416, "VISA resource name"=w411) -> ("error out"=w421:errorcluster, "Position"=w420:dbl, "VISA resource name out"=w422:refnum<visa-resource-name>)  [unwired: 7 in]
              n204 = local write "Initial Position"(w420) -> ()
              n205 = local read "Units (0: microsteps)"() -> (w425:u16)
              n206 = case shown="False" w426 {
                tunnel: w407 -> [w458 w469]
                tunnel: w425 -> [w455 w467]
                tunnel: w421 -> [w457 w465]
                tunnel: "01" ("Device and Axis") -> [w454 w464]
                tunnel: w422 -> [w460 w463]
                tunnel: [w456 w462] -> w424
                tunnel: [w459 w461] -> w423
                frame False {
                  n207 = call <instrlib>:"Move at Velocity.vi"("Units (0: device speed units)"=w455, "Velocity"=w458, "error in (no error)"=w457, "Device and Axis"=w454, "VISA resource name"=w460) -> ("error out"=w456:errorcluster, "VISA resource name out"=w459:refnum<visa-resource-name>)  [unwired: 5 in]
                }
                frame True {
                  n208 = Multiply(x=-1.0, y=w469) -> (x*y=w466:dbl)
                  n209 = call <instrlib>:"Move at Velocity.vi"("Units (0: device speed units)"=w467, "Velocity"=w466, "error in (no error)"=w465, "Device and Axis"=w464, "VISA resource name"=w463) -> ("error out"=w462:errorcluster, "VISA resource name out"=w461:refnum<visa-resource-name>)  [unwired: 5 in]
                }
              }
              n210 = local read "no of revs per velocity"() -> (w414:i32)
              n211 = property on="Revolutions Completed" class="Slide (strict)"("Scale.Maximum"=w414) -> ()  [unwired: 2 in, 2 out]
              n212 = Multiply(x=w414, y=64000.0) -> (x*y=w419:dbl)
              n213 = while {
                tunnel: [w452] -> w410
                tunnel: [w451] -> w415
                tunnel: w424 -> [w450]
                tunnel: w423 -> [w449]
                tunnel: w419 -> [w441]
                tunnel: [w448] -> _
                shift-right: [w435] -> _
                shift-left: 0 -> [w436]
                stop <- w448 stop-if-true
                # "stops when microsteps comp>=microsteps total"
                # "microsteps? completed"
                n214 = local read "STOP Rotating Motor"() -> (w453:bool)
                n215 = call <instrlib>:"Read Current Position.vi"("error in (no error)"=w450, "VISA resource name"=w449) -> ("error out"=w451:errorcluster, "Position"=w446:dbl, "VISA resource name out"=w452:refnum<visa-resource-name>)  [unwired: 7 in]
                n216 = Increment(x=w436) -> (x+1=w439:i32)
                n217 = local read "ABORT"() -> (w434:bool)
                n218 = local read "Initial Position"() -> (w445:dbl)
                n219 = local read "Track Radius (mm)"() -> (w428:T1)
                n220 = Subtract(x=w446, y=w445) -> (x-y=w432:dbl)
                n221 = Divide(x=w432, y=64000.0) -> (x/y=w430:dbl)
                n222 = Multiply(x=6.283185307179586, y=w430) -> (x*y=w429:dbl)
                n223 = Multiply(x=w439, y=64000.0) -> (x*y=w438:dbl)
                n224 = Greater Or Equal?(x=w432, y=w438) -> (x >= y?=w437:bool)
                n225 = Less Or Equal?(x=w441, y=w432) -> (x <= y?=w447:bool)
                n226 = Divide(x=w432, y=w441) -> (x/y=w444:dbl)
                n227 = Multiply(x=w429, y=w428) -> (x*y=w427:dbl)
                n228 = local write "Sliding Distance (mm)"(w427) -> ()
                n229 = Select(t=w439, s=w437, f=w436) -> (s? t:f=w435:i32)
                n230 = local write "Revolutions Completed"(w435) -> ()
                n231 = Compound Arithmetic op=OR(w447, w453, w434) -> (w448:bool)
                n232 = Multiply(x=100.0, y=w444) -> (x*y=w443:dbl)
                n233 = local write "Progress"(w443) -> ()
              }
              n234 = local read "ABORT"() -> (w412:bool)
              n235 = local read "STOP Rotating Motor"() -> (w413:bool)
              n236 = Or(x=w412, y=w413) -> (x .or. y?=w406:bool)
            }
            frame "Stop" {
              n237 = call <instrlib>:"Stop.vi"("error in (no error)"=w472, "VISA resource name"=w470) -> ("error out"=w473:errorcluster, "VISA resource name out"=w474:refnum<visa-resource-name>)  [unwired: 8 in]
              n238 = call <instrlib>:"Close.vi"("error in (no error)"=w473, "VISA resource name"=w474) -> ()  [unwired: 9 in, 1 out]
            }
          }
          n239 = Stop(stop? (T)=w386) -> ()
        }
        n240 = call "Motor speed settings.vi"("reference (in)"=w367, "HSPD"=1000, "LSPD"=1000, "ACC"=10) -> ("reference (out)"=w369:refnum<class "_Controller.lvclass">)  [unwired: 10 in, 1 out]
        n241 = call <instrlib>:"send_receive_command.vi"("reference (in)"=w369, "ASCII Command (in)"="PX=0") -> ("reference (out)"=w368:refnum<class "_Controller.lvclass">)  [unwired: 13 in, 4 out]
        n242 = while {
          tunnel: w368 -> [w486]
          tunnel: [w476] -> w366
          tunnel: w371 -> [w477]
          i -> [w484]
          stop <- w480 continue-if-true
          n243 = Dequeue Element(queue=w477) -> (element=w478:i32, error out=w479:errorcluster)  [unwired: 2 in, 2 out]
          "received P" <- w478
          n244 = call <vilib>:"Clear Errors.vi"("error in (no error)"=w479) -> ()  [unwired: 5 in, 2 out]
          n245 = call "Xn.vi"("Position"=w478, "_Controller in"=w486) -> ("_Controller out"=w485:refnum<class "_Controller.lvclass">)  [unwired: 8 in, 1 out]
          n246 = local read "Testing"() -> (w481:bool)
          n247 = local read "ABORT"() -> (w483:bool)
          n248 = control-ref of="ABORT"() -> (w475:refnum<vi>)
          n249 = call "WAIT 0.vi"("reference"=w475, "_Controller in"=w485) -> ("_Controller out"=w476:refnum<class "_Controller.lvclass">)  [unwired: 7 in, 2 out]
          n250 = Not(x=w483) -> (.not. x?=w482:bool)
          n251 = And(x=w481, y=w482) -> (x .and. y?=w480:bool)
          "Correction loop" <- w484
        }
      }
      frame "Terminate" {
        n252 = control-ref of="ABORT"() -> (w489:refnum<vi>)
        n253 = control-ref of="ABORT"() -> (w490:refnum<vi>)
        n254 = Unbundle(w499) -> (w498, w497, w496)
        n255 = call "WAIT 0.vi"("reference"=w489, "_Controller in"=w492) -> ("_Controller out"=w502:refnum<class "_Controller.lvclass">)  [unwired: 7 in, 2 out]
        n256 = call "WAIT 0.vi"("reference"=w490, "_Controller in"=w493) -> ("_Controller out"=w507:refnum<class "_Controller.lvclass">)  [unwired: 7 in, 2 out]
        n257 = case shown="False" FALSE {
          tunnel: w494 -> [w512 w529]
          tunnel: [w511 w526] -> w491
          frame False {
            n258 = call "Motor speed settings.vi"("reference (in)"=w512, "HSPD"=22000, "LSPD"=1000, "ACC"=500) -> ("reference (out)"=w517:refnum<class "_Controller.lvclass">)  [unwired: 10 in, 1 out]
            n259 = Negate(x=600 ("Position")) -> (-x=w518:i32)
            n260 = call "Xn.vi"("Position"=w518, "_Controller in"=w517) -> ("_Controller out"=w519:refnum<class "_Controller.lvclass">)  [unwired: 8 in, 1 out]
            n261 = control-ref of="ABORT"() -> (w510:refnum<vi>)
            n262 = call "WAIT 0.vi"("reference"=w510, "_Controller in"=w519) -> ("_Controller out"=w511:refnum<class "_Controller.lvclass">)  [unwired: 7 in, 2 out]
          }
          frame True {
            n263 = call "Motor speed settings.vi"("reference (in)"=w529, "HSPD"=22000, "LSPD"=1000, "ACC"=500) -> ("reference (out)"=w523:refnum<class "_Controller.lvclass">)  [unwired: 10 in, 1 out]
            n264 = Negate(x=80000 ("Position")) -> (-x=w524:i32)
            n265 = call "Xn.vi"("Position"=w524, "_Controller in"=w523) -> ("_Controller out"=w527:refnum<class "_Controller.lvclass">)  [unwired: 8 in, 1 out]
            n266 = control-ref of="ABORT"() -> (w528:refnum<vi>)
            n267 = call "WAIT 0.vi"("reference"=w528, "_Controller in"=w527) -> ("_Controller out"=w526:refnum<class "_Controller.lvclass">)  [unwired: 7 in, 2 out]
          }
        }
        n268 = Release Queue(queue=w495) -> ()  [unwired: 2 in, 3 out]
        n269 = Release Queue(queue=w496) -> ()  [unwired: 2 in, 3 out]
        n270 = call <instrlib>:"send_receive_command.vi"("reference (in)"=w502, "ASCII Command (in)"="SR0=1") -> ("reference (out)"=w503:refnum<class "_Controller.lvclass">)  [unwired: 13 in, 4 out]
        n271 = Release Queue(queue=w497) -> ()  [unwired: 2 in, 3 out]
        n272 = call <instrlib>:"send_receive_command.vi"("reference (in)"=w507, "ASCII Command (in)"="SR0=1") -> ("reference (out)"=w506:refnum<class "_Controller.lvclass">)  [unwired: 13 in, 4 out]
        n273 = Release Queue(queue=w498) -> ()  [unwired: 2 in, 3 out]
        n274 = call <instrlib>:"close_connection.vi"("reference (in)"=w503) -> ()  [unwired: 17 in, 2 out]
        n275 = call <instrlib>:"close_connection.vi"("reference (in)"=w506) -> ()  [unwired: 17 in, 2 out]
        n276 = call <instrlib>:"send_receive_command.vi"("reference (in)"=w491, "ASCII Command (in)"="SR0=1") -> ("reference (out)"=w508:refnum<class "_Controller.lvclass">)  [unwired: 13 in, 4 out]
        n277 = call <instrlib>:"close_connection.vi"("reference (in)"=w508) -> ("error out"=w488:errorcluster)  [unwired: 17 in, 1 out]
        n278 = local read "ABORT"() -> (w501:bool)
        n279 = case shown="True" w501 {
          tunnel: [w530 w531] -> w500
          tunnel: w488 -> [_ _]
          frame False {
            w530 = TRUE ("Value (Signaling)")
            n280 = property on="ABORT" class="Bool (strict)"("Val(Sgnl)"=w530) -> ()  [unwired: 2 in, 2 out]
            n281 = local write "Completed"(w530) -> ()
          }
          frame True {
            w531 = TRUE ("Value (Signaling)")
            n282 = local write "Aborted"(w531) -> ()
          }
        }
      }
    }
  }
  n283 = Format Into String(Queue_names."x-axis ref queue" ("Enum")) -> (resulting string=w18:string)  [unwired: 3 in, 1 out]
  n284 = Format Into String(Queue_names."y-axis ref queue" ("Enum")) -> (resulting string=w19:string)  [unwired: 3 in, 1 out]
  n285 = Format Into String(Queue_names."z-axis ref queue" ("Enum")) -> (resulting string=w17:string)  [unwired: 3 in, 1 out]
  n286 = Obtain Queue(name (unnamed)=w17, element data type=w3) -> (queue out=w9:refnum<queue>, error out=w8:errorcluster)  [unwired: 3 in, 1 out]
  n287 = Obtain Queue(name (unnamed)=w18, element data type=w3) -> (queue out=w11:refnum<queue>, error out=w10:errorcluster)  [unwired: 3 in, 1 out]
  n288 = Obtain Queue(name (unnamed)=w19, element data type=w3) -> (queue out=w13:refnum<queue>, error out=w12:errorcluster)  [unwired: 3 in, 1 out]
  n289 = while "Manual Control Enabling Loop" {
    tunnel: w13 -> [w547]
    tunnel: w12 -> [w546]
    tunnel: w11 -> [w545]
    tunnel: w10 -> [w544]
    tunnel: w9 -> [w543]
    tunnel: w8 -> [w542]
    tunnel: [w537] -> w7
    tunnel: [w536] -> w6
    tunnel: [w535] -> w5
    stop <- w548 stop-if-true
    n290 = Preview Queue Element(queue=w543, error in (no error)=w542) -> (queue out=w541:refnum<queue>, element=w534:refnum<class "_Controller.lvclass">)  [unwired: 1 in, 2 out]
    n291 = Preview Queue Element(queue=w545, error in (no error)=w544) -> (queue out=w540:refnum<queue>, element=w533:refnum<class "_Controller.lvclass">)  [unwired: 1 in, 2 out]
    n292 = Preview Queue Element(queue=w547, error in (no error)=w546) -> (queue out=w539:refnum<queue>, element=w532:refnum<class "_Controller.lvclass">)  [unwired: 1 in, 2 out]
    n293 = Bundle("queue out"=w541, "queue out"=w540, "queue out"=w539) -> (w538:T11)  [unwired: 1 in]
    n294 = event shown="[4] \"Left\": Value Change" {
      selector: _ -> [_ _ _ _ _ _ _ _ _ _]
      dyn-events: _ -> [_ _ _ _ _ _ _ _ _ _]
      timeout: _ -> [_ _ _ _ _ _ _ _ _ _]
      tunnel: w534 -> [_ _ w587 w598 _ _ _ _ _ _]
      tunnel: w533 -> [_ _ _ _ w609 w620 _ _ _ _]
      tunnel: w532 -> [_ _ _ _ _ _ w631 w642 _ _]
      tunnel: [_ _ _ _ _ _ _ _ _ w657] -> w548
      event Timeout {
        n295 = event-data() -> ()  [unwired: 1 in, 3 out]
      }
      event Key Down; Key Up {
        n296 = event-data() -> ("Type"=w550:T13, "ScanCode"=w551:i16)  [unwired: 1 in, 2 out]
        n297 = property on="Manual control" class="Bool (strict)"() -> ("Value"=w549:bool)  [unwired: 2 in, 2 out]
        n298 = case shown="True" w549 {
          tunnel: w551 -> [_ w553]
          tunnel: w550 -> [_ w552]
          frame False {
          }
          frame True {
            n299 = case shown="20" w553 {
              tunnel: w552 -> [_ w555 w560 w565 w570 w575 w580 w584]
              frame 0, Default {
              }
              frame 72 {
                # "Up"
                n300 = local read "Down"() -> (w554:bool)
                n301 = case shown="False" w554 {
                  tunnel: w555 -> [w556 _]
                  frame False {
                    n302 = case shown="\"Key Down\"" w556 {
                      frame "Null", Default {
                      }
                      frame "Key Down" {
                        n303 = property on="Up" class="Bool (strict)"("Val(Sgnl)"=TRUE) -> ()  [unwired: 2 in, 2 out]
                      }
                      frame "Key Up" {
                        n304 = property on="Up" class="Bool (strict)"("Val(Sgnl)"=FALSE) -> ()  [unwired: 2 in, 2 out]
                      }
                    }
                  }
                  frame True {
                  }
                }
              }
              frame 80 {
                # "Down"
                n305 = local read "Up"() -> (w559:bool)
                n306 = case shown="False" w559 {
                  tunnel: w560 -> [w561 _]
                  frame False {
                    n307 = case shown="\"Key Up\"" w561 {
                      frame "Null", Default {
                      }
                      frame "Key Down" {
                        n308 = property on="Down" class="Bool (strict)"("Val(Sgnl)"=TRUE) -> ()  [unwired: 2 in, 2 out]
                      }
                      frame "Key Up" {
                        n309 = property on="Down" class="Bool (strict)"("Val(Sgnl)"=FALSE) -> ()  [unwired: 2 in, 2 out]
                      }
                    }
                  }
                  frame True {
                  }
                }
              }
              frame 75 {
                # "Left"
                n310 = local read "Right"() -> (w564:bool)
                n311 = case shown="False" w564 {
                  tunnel: w565 -> [w566 _]
                  frame False {
                    n312 = case shown="\"Key Up\"" w566 {
                      frame "Null", Default {
                      }
                      frame "Key Down" {
                        n313 = property on="Left" class="Bool (strict)"("Val(Sgnl)"=TRUE) -> ()  [unwired: 2 in, 2 out]
                      }
                      frame "Key Up" {
                        n314 = property on="Left" class="Bool (strict)"("Val(Sgnl)"=FALSE) -> ()  [unwired: 2 in, 2 out]
                      }
                    }
                  }
                  frame True {
                  }
                }
              }
              frame 77 {
                # "Right"
                n315 = local read "Left"() -> (w569:bool)
                n316 = case shown="False" w569 {
                  tunnel: w570 -> [w571 _]
                  frame False {
                    n317 = case shown="\"Key Up\"" w571 {
                      frame "Null", Default {
                      }
                      frame "Key Down" {
                        n318 = property on="Right" class="Bool (strict)"("Val(Sgnl)"=TRUE) -> ()  [unwired: 2 in, 2 out]
                      }
                      frame "Key Up" {
                        n319 = property on="Right" class="Bool (strict)"("Val(Sgnl)"=FALSE) -> ()  [unwired: 2 in, 2 out]
                      }
                    }
                  }
                  frame True {
                  }
                }
              }
              frame 24 {
                # "Out"
                n320 = local read "In"() -> (w574:bool)
                n321 = case shown="False" w574 {
                  tunnel: w575 -> [w576 _]
                  frame False {
                    n322 = case shown="\"Key Up\"" w576 {
                      frame "Null", Default {
                      }
                      frame "Key Down" {
                        n323 = property on="Out" class="Bool (strict)"("Val(Sgnl)"=TRUE) -> ()  [unwired: 2 in, 2 out]
                      }
                      frame "Key Up" {
                        n324 = property on="Out" class="Bool (strict)"("Val(Sgnl)"=FALSE) -> ()  [unwired: 2 in, 2 out]
                      }
                    }
                  }
                  frame True {
                  }
                }
              }
              frame 23 {
                # "In"
                n325 = local read "Out"() -> (w579:bool)
                n326 = case shown="False" w579 {
                  tunnel: w580 -> [w581 _]
                  frame False {
                    n327 = case shown="\"Key Up\"" w581 {
                      frame "Null", Default {
                      }
                      frame "Key Down" {
                        n328 = property on="In" class="Bool (strict)"("Val(Sgnl)"=TRUE) -> ()  [unwired: 2 in, 2 out]
                      }
                      frame "Key Up" {
                        n329 = property on="In" class="Bool (strict)"("Val(Sgnl)"=FALSE) -> ()  [unwired: 2 in, 2 out]
                      }
                    }
                  }
                  frame True {
                  }
                }
              }
              frame 20 {
                n330 = case shown="\"Key Down\"" w584 {
                  frame "Null", Default {
                  }
                  frame "Key Down" {
                    n331 = local write "TARE"(TRUE ("TARE")) -> ()
                  }
                }
              }
            }
          }
        }
      }
      event "Up": Value Change {
        n332 = event-data() -> ()  [unwired: 1 in, 1 out]
        n333 = property on="Manual control" class="Bool (strict)"() -> ("Value"=w586:bool)  [unwired: 2 in, 2 out]
        n334 = case shown="True" w586 {
          tunnel: w587 -> [_ w588]
          frame False {
          }
          frame True {
            n335 = local read "Up"() -> (w589:bool)
            n336 = case shown="True" w589 {
              tunnel: w588 -> [w593 w596]
              frame False {
                n337 = call <instrlib>:"send_receive_command.vi"("reference (in)"=w593, "ASCII Command (in)"="STOP") -> ("reference (out)"=w591:refnum<class "_Controller.lvclass">)  [unwired: 13 in, 4 out]
                n338 = property on="Down" class="Bool (strict)"("DisabledEnum"=T6."Enabled" ("Disabled")) -> ()  [unwired: 2 in, 2 out]
                n339 = call "WAITX.vi"("_Controller in"=w591) -> ()  [unwired: 8 in, 3 out]
              }
              frame True {
                n340 = call-dynamic "jogMotor.vi"("Controller in"=w596, "dir"=linear_direction."NEG (-)") -> ()  [unwired: 14 in, 4 out]
                n341 = property on="Down" class="Bool (strict)"("DisabledEnum"=T6."Disabled" ("Disabled")) -> ()  [unwired: 2 in, 2 out]
              }
            }
          }
        }
      }
      event "Down": Value Change {
        n342 = event-data() -> ()  [unwired: 1 in, 1 out]
        n343 = property on="Manual control" class="Bool (strict)"() -> ("Value"=w597:bool)  [unwired: 2 in, 2 out]
        n344 = case shown="True" w597 {
          tunnel: w598 -> [_ w600]
          frame False {
          }
          frame True {
            n345 = local read "Down"() -> (w599:bool)
            n346 = case shown="True" w599 {
              tunnel: w600 -> [w604 w607]
              frame False {
                n347 = call <instrlib>:"send_receive_command.vi"("reference (in)"=w604, "ASCII Command (in)"="STOP") -> ("reference (out)"=w602:refnum<class "_Controller.lvclass">)  [unwired: 13 in, 4 out]
                n348 = property on="Up" class="Bool (strict)"("DisabledEnum"=T6."Enabled" ("Disabled")) -> ()  [unwired: 2 in, 2 out]
                n349 = call "WAITX.vi"("_Controller in"=w602) -> ()  [unwired: 8 in, 3 out]
              }
              frame True {
                n350 = call-dynamic "jogMotor.vi"("Controller in"=w607, "dir"=linear_direction."POS (+)") -> ()  [unwired: 14 in, 4 out]
                n351 = property on="Up" class="Bool (strict)"("DisabledEnum"=T6."Disabled" ("Disabled")) -> ()  [unwired: 2 in, 2 out]
              }
            }
          }
        }
      }
      event "Left": Value Change {
        n352 = event-data() -> ()  [unwired: 1 in, 1 out]
        n353 = property on="Manual control" class="Bool (strict)"() -> ("Value"=w608:bool)  [unwired: 2 in, 2 out]
        n354 = case shown="True" w608 {
          tunnel: w609 -> [_ w611]
          frame False {
          }
          frame True {
            n355 = local read "Left"() -> (w610:bool)
            n356 = case shown="True" w610 {
              tunnel: w611 -> [w615 w618]
              frame False {
                n357 = call <instrlib>:"send_receive_command.vi"("reference (in)"=w615, "ASCII Command (in)"="STOP") -> ("reference (out)"=w613:refnum<class "_Controller.lvclass">)  [unwired: 13 in, 4 out]
                n358 = call "WAITX.vi"("_Controller in"=w613) -> ()  [unwired: 8 in, 3 out]
                n359 = property on="Right" class="Bool (strict)"("DisabledEnum"=T6."Enabled" ("Disabled")) -> ()  [unwired: 2 in, 2 out]
              }
              frame True {
                n360 = call-dynamic "jogMotor.vi"("Controller in"=w618, "dir"=linear_direction."NEG (-)") -> ()  [unwired: 14 in, 4 out]
                n361 = property on="Right" class="Bool (strict)"("DisabledEnum"=T6."Disabled" ("Disabled")) -> ()  [unwired: 2 in, 2 out]
              }
            }
          }
        }
      }
      event "Right": Value Change {
        n362 = event-data() -> ()  [unwired: 1 in, 1 out]
        n363 = property on="Manual control" class="Bool (strict)"() -> ("Value"=w619:bool)  [unwired: 2 in, 2 out]
        n364 = case shown="True" w619 {
          tunnel: w620 -> [_ w622]
          frame False {
          }
          frame True {
            n365 = local read "Right"() -> (w621:bool)
            n366 = case shown="False" w621 {
              tunnel: w622 -> [w626 w629]
              frame False {
                n367 = call <instrlib>:"send_receive_command.vi"("reference (in)"=w626, "ASCII Command (in)"="STOP") -> ("reference (out)"=w624:refnum<class "_Controller.lvclass">)  [unwired: 13 in, 4 out]
                n368 = call "WAITX.vi"("_Controller in"=w624) -> ()  [unwired: 8 in, 3 out]
                n369 = property on="Left" class="Bool (strict)"("DisabledEnum"=T6."Enabled" ("Disabled")) -> ()  [unwired: 2 in, 2 out]
              }
              frame True {
                n370 = call-dynamic "jogMotor.vi"("Controller in"=w629, "dir"=linear_direction."POS (+)") -> ()  [unwired: 14 in, 4 out]
                n371 = property on="Left" class="Bool (strict)"("DisabledEnum"=T6."Disabled" ("Disabled")) -> ()  [unwired: 2 in, 2 out]
              }
            }
          }
        }
      }
      event "Out": Value Change {
        n372 = event-data() -> ()  [unwired: 1 in, 1 out]
        n373 = property on="Manual control" class="Bool (strict)"() -> ("Value"=w630:bool)  [unwired: 2 in, 2 out]
        n374 = case shown="True" w630 {
          tunnel: w631 -> [_ w633]
          frame False {
          }
          frame True {
            n375 = local read "Out"() -> (w632:bool)
            n376 = case shown="True" w632 {
              tunnel: w633 -> [w637 w640]
              frame False {
                n377 = call <instrlib>:"send_receive_command.vi"("reference (in)"=w637, "ASCII Command (in)"="STOP") -> ("reference (out)"=w635:refnum<class "_Controller.lvclass">)  [unwired: 13 in, 4 out]
                n378 = property on="In" class="Bool (strict)"("DisabledEnum"=T6."Enabled" ("Disabled")) -> ()  [unwired: 2 in, 2 out]
                n379 = call "WAITX.vi"("_Controller in"=w635) -> ()  [unwired: 8 in, 3 out]
              }
              frame True {
                n380 = call-dynamic "jogMotor.vi"("Controller in"=w640, "dir"=linear_direction."NEG (-)") -> ()  [unwired: 14 in, 4 out]
                n381 = property on="In" class="Bool (strict)"("DisabledEnum"=T6."Disabled" ("Disabled")) -> ()  [unwired: 2 in, 2 out]
              }
            }
          }
        }
      }
      event "In": Value Change {
        n382 = event-data() -> ()  [unwired: 1 in, 1 out]
        n383 = property on="Manual control" class="Bool (strict)"() -> ("Value"=w641:bool)  [unwired: 2 in, 2 out]
        n384 = case shown="True" w641 {
          tunnel: w642 -> [_ w644]
          frame False {
          }
          frame True {
            n385 = local read "In"() -> (w643:bool)
            n386 = case shown="True" w643 {
              tunnel: w644 -> [w648 w649]
              frame False {
                n387 = call <instrlib>:"send_receive_command.vi"("reference (in)"=w648, "ASCII Command (in)"="STOP") -> ("reference (out)"=w646:refnum<class "_Controller.lvclass">)  [unwired: 13 in, 4 out]
                n388 = call "WAITX.vi"("_Controller in"=w646) -> ()  [unwired: 8 in, 3 out]
                n389 = property on="Out" class="Bool (strict)"("DisabledEnum"=T6."Enabled" ("Disabled")) -> ()  [unwired: 2 in, 2 out]
              }
              frame True {
                n390 = call-dynamic "jogMotor.vi"("Controller in"=w649, "dir"=linear_direction."POS (+)") -> ()  [unwired: 14 in, 4 out]
                n391 = property on="Out" class="Bool (strict)"("DisabledEnum"=T6."Disabled" ("Disabled")) -> ()  [unwired: 2 in, 2 out]
              }
            }
          }
        }
      }
      event "Approach": Value Change {
        n392 = event-data() -> ()  [unwired: 1 in, 1 out]
        n393 = local read "Manual control"() -> (w652:bool)
        n394 = case shown="True" w652 {
          frame False {
          }
          frame True {
            n395 = local read "Approach"() -> (w653:bool)
            n396 = case shown="False" w653 {
              frame False {
              }
              frame True {
                n397 = flat-sequence {
                  tunnel: [FALSE ("Approach")] -> w654
                  frame #0 {
                    n398 = Wait Until Next ms Multiple(millisecond multiple=u32 300) -> ()  [unwired: 1 out]
                  }
                }
                n399 = local write "Approach"(w654) -> ()
              }
            }
          }
        }
      }
      event "ABORT": Value Change {
        n400 = event-data() -> ()  [unwired: 1 in, 1 out]
        n401 = local read "ABORT"() -> (w658:bool)
        n402 = case shown="False" w658 {
          tunnel: [FALSE TRUE] -> w657
          frame False {
          }
          frame True {
          }
        }
      }
    }
    n403 = Unbundle(w538) -> ("queue out"=w537:refnum<queue>, "queue out"=w536:refnum<queue>, "queue out"=w535:refnum<queue>)
  }
  n404 = Release Queue(queue=w7) -> ()  [unwired: 2 in, 3 out]
  n405 = Release Queue(queue=w6) -> ()  [unwired: 2 in, 3 out]
  n406 = Release Queue(queue=w5) -> ()  [unwired: 2 in, 3 out]
  n407 = while "Logic Loop" {
    shift-right: [w666] -> _
    shift-left: Logic_states."Initialize" ("Enum") -> [w667]
    shift-right: [w664] -> _
    shift-left: _ -> [w663]
    shift-right: [w662] -> _
    shift-left: _ -> [w661]
    stop <- w665 stop-if-true
    n408 = case shown="\"Process\"" w667 {
      tunnel: [w672 Logic_states."Terminate" ("Enum") _] -> w666
      tunnel: [_ _ TRUE] -> w665
      tunnel: [w681 w743 _] -> w664
      tunnel: w663 -> [_ w743 w856]
      tunnel: [w669 _ _] -> w662
      tunnel: w661 -> [_ w717 _]
      frame "Initialize", Default {
        n409 = call <vilib>:"Check if File or Folder Exists.vi"("path"="Save file name") -> ("file or folder exists?"=w679:bool, "dup path"=w678:path)  [unwired: 8 in, 1 out]
        n410 = case shown="True" w679 {
          tunnel: w678 -> [w706 w709]
          tunnel: [TRUE ("T button?") w714] -> w676
          tunnel: [w706 w709] -> w677
          tunnel: [FALSE w713] -> w673
          frame False {
          }
          frame True {
            n411 = Strip Path(path=w709) -> (name=w708:string)  [unwired: 1 out]
            n412 = Concatenate Strings("Warning!\nThis File already exists: " ("message"), "\r", w708) -> (w710:string)
            n413 = Two Button Dialog(message=w710, 1:"Abort" ("F button name (\"Cancel\")"), 2:"Overwrite" ("T button name (\"OK\")")) -> (T button?=w714:bool)
            n414 = Not(x=w714) -> (.not. x?=w713:bool)
            n415 = property on="ABORT" class="Bool (strict)"("Val(Sgnl)"=w713) -> ()  [unwired: 2 in, 2 out]
          }
        }
        n416 = case shown="True" w676 {
          tunnel: w677 -> [_ w704]
          tunnel: [_ w689] -> w669
          frame False {
          }
          frame True {
            n417 = local read "Sampling frequency (rate)"() -> (w698:T1)
            n418 = local read "Track Radius (mm)"() -> (w696:T1)
            n419 = local read "Steady State COFs"() -> (w685:dbl[])
            n420 = local read "Velocity"() -> (w697:dbl)
            n421 = local read "Wear cycles"() -> (w695:i32)
            n422 = Number To Decimal String(number=w698) -> (decimal integer string=w694:string)  [unwired: 1 in]
            n423 = Number To Decimal String(number=w697) -> (decimal integer string=w693:string)  [unwired: 1 in]
            n424 = Number To Decimal String(number=w696) -> (decimal integer string=w692:string)  [unwired: 1 in]
            n425 = Number To Decimal String(number=w695) -> (decimal integer string=w691:string)  [unwired: 1 in]
            n426 = Number To Decimal String(number=w685) -> (decimal integer string=w684:string[])  [unwired: 1 in]
            n427 = Build Array (concatenate)("Sampling fequency [Hz]:", w694, "Velocity [microsteps]: ", w693, "Track radius [mm]:", w692, "Cycles:", w691, "Steady State COFs:", w684) -> (w690:string[])
            n428 = call-poly <vilib>:"Write Delimited Spreadsheet.vi"("file path (dialog if empty)"=w704, "1D data"=w690) -> ("new file path (Not A Path if cancelled)"=w703:path)  [unwired: 12 in, 1 out]
            n429 = call-poly <vilib>:"Write Delimited Spreadsheet.vi"("file path (dialog if empty)"=w703, "1D data"=string[] ["Fx", "Fy", "Fz", "Tx", "Ty", "Tz", "Angular Position"], "append to file? (new file:F)"=TRUE) -> ("new file path (Not A Path if cancelled)"=w689:path)  [unwired: 11 in, 1 out]
          }
        }
        n430 = Format Into String(Queue_names."Cell queue name" ("Enum")) -> (resulting string=w670:string)  [unwired: 3 in, 1 out]
        n431 = Obtain Queue(name (unnamed)=w670, element data type=dbl[] []) -> (queue out=w682:refnum<queue>, error out=w680:errorcluster)  [unwired: 3 in, 1 out]
        n432 = Bundle("queue out"=w682, "error out"=w680) -> (w681:T7)  [unwired: 1 in]
        n433 = Select(t=Logic_states."Terminate" ("Enum"), s=w673, f=Logic_states."Process" ("Enum")) -> (s? t:f=w672:T5)
      }
      frame "Process" {
        n434 = Unbundle(w743) -> ("queue out"=w720:refnum<queue>, "error out"=w719:errorcluster)
        n435 = local read "Sampling frequency (rate)"() -> (w740:T1)
        n436 = while "Saving Data" {
          tunnel: w717 -> [w840]
          tunnel: w720 -> [w839]
          tunnel: w719 -> [w838]
          stop <- w846 stop-if-true
          w843 = u16 2 items=["x-load", "y-load", "z-load", "x-torque", "y-torque", "z-torque"]
          n437 = Flush Queue(queue=w839, error in (no error)=w838) -> (remaining elements=w844:cluster{dbl[]}[])  [unwired: 2 out]
          n438 = for {
            tunnel: w844 -> [w849] mode=indexing
            tunnel: [w848] -> w842 mode=indexing
            n439 = Unbundle(w849) -> (w848:dbl[])
          }
          n440 = call-poly <vilib>:"Write Delimited Spreadsheet.vi"("file path (dialog if empty)"=w840, "2D data"=w842, "append to file? (new file:F)"=TRUE) -> ()  [unwired: 11 in, 2 out]
          n441 = Index Array(array=w842, index (col)=w843) -> (element=w841:dbl[])  [unwired: 1 in]
          n442 = Negate(x=w841) -> (-x=→"Dequeued Data":dbl[])
          n443 = local read "ABORT"() -> (w846:bool)
        }
        n444 = Less Or Equal?(x=w740, y=u16 50) -> (x <= y?=w742:bool)
        n445 = Reciprocal(x=w740) -> (1/x=w739:dbl)
        n446 = Multiply(x=1000.0, y=w739) -> (x*y=w737:dbl)
        n447 = Format Into String(Queue_names."Feedback" ("Enum")) -> (resulting string=w723:string)  [unwired: 3 in, 1 out]
        n448 = Select(t=w737, s=w742, f=10.0) -> (s? t:f=w728:dbl)
        n449 = Divide(x=w728, y=1000.0) -> (x/y=w729:dbl)
        n450 = Obtain Queue(max queue size (-1, unlimited)=1, name (unnamed)=w723, element data type=0) -> (queue out=w722:refnum<queue>)  [unwired: 2 in, 2 out]
        n451 = Format Into String(Queue_names."to PID" ("Enum")) -> (resulting string=w733:string)  [unwired: 3 in, 1 out]
        n452 = Obtain Queue(max queue size (-1, unlimited)=1, name (unnamed)=w733, element data type=0.0) -> (queue out=w730:refnum<queue>)  [unwired: 2 in, 2 out]
        n453 = while "Averaging" {
          tunnel: w728 -> [w799]
          tunnel: w730 -> [w784]
          tunnel: [w774] -> w718
          tunnel: w717 -> [w769]
          stop <- w801 stop-if-true
          w782 = u16 5 items=["x-load", "y-load", "z-load", "x-torque", "y-torque", "z-torque"]
          w798 = u16 5 items=["x-load", "y-load", "z-load", "x-torque", "y-torque", "z-torque"]
          w804 = u16 2 items=["x-load", "y-load", "z-load", "x-torque", "y-torque", "z-torque"]
          n454 = local read "Number of Previous Points"() -> (w773:i32)
          n455 = local read "Current reading"() -> (w777:dbl[])
          n456 = Wait (ms)(milliseconds to wait=w799) -> ()  [unwired: 1 out]
          n457 = local read "Track Radius (mm)"() -> (w779:T1)
          n458 = Index Array(array=w777, index=w782) -> (element=→"Torque":dbl)
          n459 = Index Array(array=w777, index=w804) -> (element=w805:dbl)
          n460 = Index Array(array=w777, index=w798) -> (element=w780:dbl)
          n461 = Negate(x=w805) -> (-x=w802:dbl)
          n462 = local read "Averaging Level"() -> (w800:i32)
          n463 = Divide(x=w780, y=w779) -> (x/y=w778:dbl)
          n464 = control-ref of="Mean z"() -> (w803:refnum<vi>)
          n465 = local read "Averaging Level"() -> (w796:i32)
          n466 = control-ref of="Mean Force from Torque"() -> (w797:refnum<vi>)
          n467 = call "Smoothing.vi"("Averaging Level"=w800, "Input reading"=w802, "Array in"=w803) -> ("mean"=w783:dbl)  [unwired: 8 in]
          "Smooth z" <- w783
          "Actual Load" <- w783
          n468 = call "Smoothing.vi"("Averaging Level"=w796, "Input reading"=w778, "Array in"=w797) -> ("mean"=w795:dbl)  [unwired: 8 in]
          "Smooth Force from Torque" <- w795
          n469 = local read "Testing Load [N]"() -> (w794:dbl)
          n470 = local read "Manual control"() -> (w791:bool)
          n471 = local read "ABORT"() -> (w785:bool)
          n472 = Divide(x=w795, y=w783) -> (x/y=w775:dbl)
          "Estimated friction coefficient" <- w775
          n473 = Greater Or Equal?(x=w783, y=w794) -> (x >= y?=w793:bool)
          n474 = Not(x=w791) -> (.not. x?=w790:bool)
          n475 = And(x=w793, y=w790) -> (x .and. y?=w792:bool)
          n476 = Greater?(x=w783, y=33.0) -> (0:w788:bool)
          n477 = Or(x=w792, y=w785) -> (x .or. y?=w786:bool)
          n478 = local read "Number of Previous Points"() -> (w776:i32)
          n479 = control-ref of="Mean Estimated Friction Coefficient"() -> (w767:refnum<vi>)
          n480 = local read "Steady State COFs"() -> (w766:dbl[])
          n481 = call "Smoothing.vi"("Averaging Level"=w776, "Input reading"=w775, "Array in"=w767) -> ("mean"=w768:dbl)  [unwired: 8 in]
          n482 = And(x=w788, y=w790) -> (x .and. y?=w787:bool)
          n483 = Build Array (concatenate)(w766, w768) -> (w770:dbl[])
          n484 = Array Size(array=w770) -> (size(s)=w772:i32)
          n485 = Greater?(x=w772, y=w773) -> (0:w771:bool)
          n486 = case shown="True" w771 {
            tunnel: w770 -> [_ w807]
            tunnel: w769 -> [_ w806]
            frame False {
            }
            frame True {
              n487 = while {
                tunnel: w806 -> [w814]
                tunnel: w807 -> [w810]
                stop <- w809 stop-if-true
                n488 = local read "Number of Previous Points"() -> (w816:i32)
                n489 = Array Size(array=w810) -> (size(s)=w821:i32)
                n490 = Decrement(x=w821) -> (x-1=w820:i32)
                n491 = Subtract(x=w820, y=w816) -> (x-y=w819:i32)
                n492 = Array Size(array=w810) -> (size(s)=w825:i32)
                n493 = Decrement(x=w825) -> (x-1=w824:i32)
                n494 = Array Subset(array=w810, index=w819, length=w816) -> (w818:dbl[])
                n495 = Index Array(array=w810, index=w824) -> (element=w811:dbl)
                n496 = local read "Maximum COF Difference"() -> (w826:i32)
                n497 = Add Array Elements(numeric array=w818) -> (sum=w817:dbl)
                n498 = Divide(x=w817, y=w816) -> (x/y=w815:dbl)
                n499 = Subtract(x=w811, y=w815) -> (x-y=w823:dbl)
                n500 = Absolute Value(x=w823) -> (abs(x)=w822:dbl)
                n501 = Greater Or Equal?(x=w822, y=w826) -> (x >= y?=w812:bool)
                n502 = while {
                  shift-right: [w828] -> _
                  shift-left: dbl[] [] -> [w830]
                  tunnel: w812 -> [w831]
                  tunnel: w811 -> [w829]
                  tunnel: [w828] -> w808
                  stop <- w827 stop-if-true
                  n503 = case shown="False" w831 {
                    tunnel: w830 -> [w832 w835]
                    tunnel: w829 -> [_ w834]
                    tunnel: [w832 w833] -> w828
                    frame False {
                    }
                    frame True {
                      n504 = Build Array (concatenate)(w835, w834) -> (w833:dbl[])
                    }
                  }
                  n505 = local read "ABORT"() -> (w827:bool)
                }
                n506 = call-poly <vilib>:"Write Delimited Spreadsheet.vi"("file path (dialog if empty)"=w814, "1D data"=w808) -> ()  [unwired: 12 in, 2 out]
                n507 = local read "ABORT"() -> (w809:bool)
                n508 = local write "Steady State COFs"(w808) -> ()
              }
            }
          }
          n509 = case shown="False" w786 {
            frame False {
            }
            frame True {
              n510 = local write "Approaching"(FALSE ("Approaching")) -> ()
            }
          }
          n511 = Lossy Enqueue Element(queue=w784, element=w783) -> (queue out=w774:refnum<queue>)  [unwired: 1 in, 3 out]
          n512 = case shown="False" w787 {
            frame False {
            }
            frame True {
              n513 = property on="ABORT" class="Bool (strict)"("Val(Sgnl)"=TRUE ("Value (Signaling)")) -> ()  [unwired: 2 in, 2 out]
            }
          }
          n514 = local read "ABORT"() -> (w801:bool)
        }
        n515 = while "PID" {
          tunnel: w729 -> [w750]
          tunnel: w730 -> [w747]
          tunnel: w722 -> [w746]
          tunnel: [w745] -> w721
          i -> [w748]
          stop <- w749 stop-if-true
          n516 = local read "Testing"() -> (w744:bool)
          n517 = case shown="True" w744 {
            tunnel: w750 -> [_ _]
            tunnel: w747 -> [_ w764]
            tunnel: w746 -> [w752 w760]
            tunnel: [w752 w759] -> w745
            frame False {
              n518 = Wait (ms)(milliseconds to wait=u32 250) -> ()  [unwired: 1 out]
            }
            frame True {
              n519 = Dequeue Element(queue=w764) -> (element=w756:dbl, error out=w761:errorcluster)  [unwired: 2 in, 2 out]
              n520 = call <vilib>:"Clear Errors.vi"("error in (no error)"=w761) -> ()  [unwired: 5 in, 2 out]
              n521 = local read "Testing Load [N]"() -> (w757:dbl)
              n522 = call-poly <vilib>:"PID.vi"("output range"="output range", "PID gains"="PID gains", "process variable"=w756, "setpoint"=w757) -> ("dt out (s)"=→"dt out (s)":dbl, "output"=w763:dbl)  [unwired: 6 in]
              "Correction [N]" <- w763
              n523 = Quotient & Remainder(x=w763, y=0.015) -> (floor(x/y)=w755:dbl)  [unwired: 1 out]
              "correction [p]" <- w755
              n524 = To Long Integer(number=w755) -> (32bit integer=w758:i32)
              n525 = Lossy Enqueue Element(queue=w760, element=w758) -> (queue out=w759:refnum<queue>)  [unwired: 1 in, 3 out]
            }
          }
          n526 = local read "ABORT"() -> (w749:bool)
          "to PID" <- w748
        }
        n527 = Release Queue(queue=w721) -> ()  [unwired: 2 in, 3 out]
        n528 = Release Queue(queue=w718) -> ()  [unwired: 2 in, 3 out]
      }
      frame "Terminate" {
        n529 = Initialize Array(0.0 ("element")) -> (w852:dbl[])  [unwired: 1 in]
        n530 = Initialize Array(0.0 ("element")) -> (w853:dbl[])  [unwired: 1 in]
        n531 = Unbundle(w856) -> ("queue out"=w855:refnum<queue>, "error out"=w854:errorcluster)
        n532 = local write "Mean Force from Torque"(w853) -> ()
        n533 = local write "Mean z"(w852) -> ()
        n534 = Release Queue(queue=w855, error in (no error)=w854) -> ()  [unwired: 1 in, 3 out]
      }
    }
  }
  "x-position" <- 0 ("x-position")
  "Angular Position" <- 0.0 ("Angular Position")
  "n" <- 1.0
